vi "Dryer Start Stop.vi"() -> ()   [LabVIEW 2016]
uses:
  Type Definitions/WILT Dryer Status Ctrl.ctl
  Type Definitions/WILT Start Stop Data.ctl
  Type Definitions/WILT Dryer Com Port Info.ctl
  Globals/Globals SS.vi
  <vilib>/Utility/file.llb/Write To Spreadsheet File (string).vi
  <vilib>/DAQmx/create/channels.llb/DAQmx Create Channel (DO-Digital Output).vi
  <vilib>/DAQmx/write.llb/DAQmx Write (Digital U32 1Chan 1Samp).vi
  <vilib>/Utility/file.llb/Write To Spreadsheet File (DBL).vi
  <vilib>/DAQmx/configure/timing.llb/DAQmx Timing (Sample Clock).vi
  <vilib>/DAQmx/create/channels.llb/DAQmx Create Channel (AI-Voltage-Basic).vi
  <vilib>/Utility/file.llb/Read From Spreadsheet File (DBL).vi
  <vilib>/DAQmx/read.llb/DAQmx Read (Analog 2D DBL NChan NSamp).vi
panel:
  in  "Tab Control":T1(tab)=enum."Raw Data"
  in  "D Data 2":dbl[](array[numeric])=[0.06788055309111314, 0.06788055309111314, 0.06788055309111314, 0.06788055309111314, 0.06788055309111314, 0.06788055309111314, 0.06788055309111314, 0.06788055309111314, 0.06788055309111314, 0.06788055309111314, 0.06788055309111314, 0.06788055309111314, 0.06788055309111314, 0.06788055309111314, 0.06788055309111314]
  in  "A Data 2":dbl[](array[numeric])
  in  "A Data":dbl[](array[numeric])
  in  "B Data":dbl[](array[numeric])
  in  "B Data 2":dbl[](array[numeric])
  in  "C Data 2":dbl[](array[numeric])
  in  "C Data":dbl[](array[numeric])
  in  "D Data":dbl[](array[numeric])=[5.851428694297497, 3.661927497414327, 3.661927497414327, 3.661927497414327, 3.661927497414327, 3.661927497414327, 3.661927497414327, 3.661927497414327, 3.661927497414327, 0.6577281807606751, 0.09762322341846881, 0.09762322341846881, 0.09762322341846881, 0.09762322341846881, 0.09762322341846881]
  in  "A save":dbl[](array[numeric])
  in  "C save":dbl[](array[numeric])
  in  "B save":dbl[](array[numeric])
  in  "D save":dbl[](array[numeric])=[5.851428694297497, 3.661927497414327, 3.661927497414327, 3.661927497414327, 3.661927497414327, 3.661927497414327, 3.661927497414327, 3.661927497414327, 3.661927497414327, 0.6577281807606751, 0.09762322341846881, 0.09762322341846881, 0.09762322341846881, 0.09762322341846881, 0.09762322341846881]
  out "Waveform Chart":dbl(graph)=0.09762322341846881
  in  "Channel":i32=6
  out "Currents":dbl[](array[numeric])=[0.0012165306634386985, -0.006587335189708488, 0.00045533310115012174, 0.009590983127054642, 0.09094609304713201, 0.048033305281516, 0.09762322341846881, 0.06788055309111314] format="%0.2f"
  in  "AI Task":refnum<k21>
  in  "Maximum Value":dbl=10.0 format="%0.2f"
  in  "Minimum Value":dbl=-10.0 format="%0.2f"
  in  "Rate":dbl=2.0 caption="Sample Rate (Hz)" format="%0.2f"
  in  "Samples per Channel":i32=1
  out "data":dbl[][](array[numeric])=[[0.0002433061326877397], [-0.0013174670379416976], [9.106662023002435e-05], [0.0019181966254109284], [0.018189218609426402], [0.0096066610563032], [0.019524644683693762], [0.013576110618222628]] format="%0.2f"
  in  "AI Channel":string="Dev2/ai0:7"
  out "Current State":string="Exit"
  out "Saving":errorcluster
  out "Stop":bool=TRUE
  out "Read Serial Count":dbl=792.0
  out "Log Coms Array":string[](array[string])=["COM2,3/1/2012,10:47:12 AM,No Com", "COM3,3/1/2012,10:47:12 AM,No Com", "COM4,3/1/2012,10:47:12 AM,No Com", "COM5,3/1/2012,10:47:12 AM,"]
  out "Status Array Out":T2[](array[typedef])=[{"Color"=0, "Last Read Status"=enum."Err", "Command:Data"="No Com", "Com Port"=2, "Time(S)"=158.546875, "Err Count"=233}, {"Color"=0, "Last Read Status"=enum."Err", "Command:Data"="No Com", "Com Port"=3, "Time(S)"=158.546875, "Err Count"=233}, {"Color"=0, "Last Read Status"=enum."Err", "Command:Data"="No Com", "Com Port"=4, "Time(S)"=158.5625, "Err Count"=233}, {"Color"=6618880, "Last Read Status"=enum."Cycle Running", "Command:Data"="", "Com Port"=5, "Time(S)"=158.5625, "Err Count"=1}]
  out "Rising Edge Out":bool[](array[boolean])
  in  "Power":bool[](array[boolean])=[FALSE, FALSE, FALSE, FALSE]
  in  "Power Port":tag="Dev2/port0" caption="Port"
  out "Restart Err Count":dbl=1.0
  in  "Cycle Save Multiple":i16=25
  out "Com Er Mess":string="Send Restart"
  out "Label Com Array":string[][](array[string])=[["Dryer A", "2"], ["Dryer B", "3"], ["Dryer C", "4"], ["Dryer D", "5"]]
  out "Current Filename":path=path "C:/Data/20120301_10_CONWAY-E5500.appl.ge.com_Dryer A_SS_Data.csv"
  in  "Timeout":i32=500
  in  "Config File":path=path "C:/data/SS_Config.ini"
  in  "Save File Path":path=path "C:/Data/Start Stop"
  out "robo?":bool
  out "Computer Name":string="CONWAY-E5500.appl.ge.com"
  in  "Cycle Count Path":path=path "c:/Data/CycleCount.csv"
  in  "Backup Hour":string="4"
  in  "Up Lim":dbl[](array[numeric])=[50.0, 50.0, 50.0, 50.0, 50.0, 4.4, 4.4, 50.0, 50.0, 50.0, 50.0, 1.0, 1.0, 1.0, 50.0, 50.0, 50.0, 50.0, 50.0, 50.0, 27.0, 27.0, 27.0, 27.0, 27.0, 27.0, 27.0, 27.0, 1.0, 1.0, 1.0, 1.0]
  in  "Low Lim 2":dbl[](array[numeric])=[-1.0, -1.0, -1.0, -1.0, -1.0, 3.5, 3.5, -1.0, -1.0, -1.0, -1.0, -1.0, -1.0, -1.0, -1.0, -1.0, -1.0, -1.0, -1.0, -1.0, -1.0, -1.0, -1.0, 22.0, -1.0, -1.0, -1.0, -1.0, -1.0, -1.0, -1.0, -1.0]
  in  "Low Lim":dbl[](array[numeric])=[-1.0, -1.0, -1.0, -1.0, -1.0, 3.5, 3.5, -1.0, -1.0, -1.0, -1.0, -1.0, -1.0, -1.0, -1.0, -1.0, -1.0, -1.0, -1.0, -1.0, -1.0, -1.0, 22.0, -1.0, -1.0, -1.0, -1.0, -1.0, -1.0, -1.0, -1.0, -1.0]
  in  "Off On Threshold":dbl=1.0
  in  "Filename Currents":path=path "c:/Data/Currents.csv"
  out "Max Len":i32
  out "A Array":string[][](array[string])
  out "B Array":string[][](array[string])
  out "D Array":string[][](array[string])=[["Dryer D,COM5,3/1/2012,10:46:45 AM,0x72:0x03\r0x72:0x03\r\nInner Coil OFF\r\nOuter Coil Relay OFF\r\nMachine EOCStep ID: 0006\r\n\r\nDrum Relay OFFCF Switch:0000"], [""], [""], [""], [""], [""], [""], ["Dryer D,COM5,3/1/2012,10:46:49 AM,0x72:0x01\r0x72:0x01\r\nMachine RunElec HS - Inlet Set Point 1 : 0330\r\nElec HS - Outlet Set Point 1 : 0135\r\nElec HS - Inlet Set Point 2: 0000\r\nElec HS - Outlet Set Point 2 : 0000\r\nElec HS - Inlet Set Point 3: 0350\r\nElec HS - Outlet Set Point 3 : 0140\r\n\r\nCurrent primitive: TimeDryStep ID: 0002\r\nBase Cycle Index: 0006\r\nEst Cycle Time In Min: 0001\r\n\r\nStart Tumble\r\nTumble"], ["Dryer D,COM5,3/1/2012,10:46:49 AM,StepID:0000\r\nCWDuration:0005\r\nStartDrum\r\nReverse Tumble set for CW\r\nDrum Relay ON\r\nCF Switch:0001\r\nDrum Started Ack\r\n1022  7113  0093  0138\r\nHtr Inh = 0004"], [""], ["Dryer D,COM5,3/1/2012,10:46:50 AM,1023  7113  0093  0138"], [""], ["Dryer D,COM5,3/1/2012,10:46:51 AM,1023  7113  0093  0138"], [""], ["Dryer D,COM5,3/1/2012,10:46:52 AM,1022  7113  0093  0139\r\n\r\nHeaterOffDuration:0000\r\nTumbleStepID:0001\r\nDrum Relay OFFReverse Tumble set for CCW"], ["Dryer D,COM5,3/1/2012,10:46:53 AM,CF Switch:0000"], ["Dryer D,COM5,3/1/2012,10:46:54 AM,1020  7113  0092  0139\r\n\r\nDrum Stop Ack\r\nCW Pause Duraiton:3000\r\nTumble Pause"], ["Dryer D,COM5,3/1/2012,10:46:54 AM,1022  7113  0092  0139"], [""], ["Dryer D,COM5,3/1/2012,10:46:55 AM,1022  7113  0093  0138"], [""], ["Dryer D,COM5,3/1/2012,10:46:56 AM,1023  7113  0093  0139\r\n\r\nTumbleStepID:0002\r\nCCWDurat"], ["Dryer D,COM5,3/1/2012,10:46:57 AM,ion:0005\r\nStartDrum\r\nDrum Relay ON\r\nCF Switch:0001"], ["Dryer D,COM5,3/1/2012,10:46:57 AM,1020  7113  0093  0139\r\nDrum Started Ack"], [""], ["Dryer D,COM5,3/1/2012,10:46:59 AM,1019  7113  0093  0139\r\nHtr Inh = 0000\r\nOuter Coil ON\r\nInner Coil ON"], ["Dryer D,COM5,3/1/2012,10:46:59 AM,1023  7113  0093  0139\r\nER1-ON \r\nER2-ON"], [""], ["Dryer D,COM5,3/1/2012,10:47:00 AM,1023  7113  0093  0139\r\n\r0x72:0x03\r0x72:0x03\r\nInner Coil OFF\r\nOuter Coil"], ["Dryer D,COM5,3/1/2012,10:47:01 AM,Relay OFF\r\nMachine EOCStep ID: 0006\r\n\r\nDrum Relay OFFCF Switch:0000"], [""], [""], [""], [""], [""], [""], ["Dryer D,COM5,3/1/2012,10:47:05 AM,0x72:0x01\r0x72:0x01\r\nMachine RunElec HS - Inlet  Outlet Set Point 1 : 0135\r\nElec HS - Inlet Set Point 2: 0000\r\nElec HS - Outlet Set Point 2 : 0000\r\nElec HS - Inlet Set Point 3: 0350\r\nElec HS - Outlet Set Point 3 : 0140\r\n\r\nCurrent primitive: TimeDryStep ID: 0002\r\nBase Cycle Index: 0006\r\nEst Cycle Time In Min: 0001\r\n\r\nStart Tumble\r\nTumbleStepID:0000\r\nCWDuration:0005"], ["Dryer D,COM5,3/1/2012,10:47:05 AM,t for CW\r\nDrum Relay ON\r\nCF Switch:0001\r\nDrum Started Ack\r\n1023  7113  0093  0139\r\nHtr Inh = 0004"], [""], ["Dryer D,COM5,3/1/2012,10:47:06 AM,1019  7113  0093  0139"], ["Dryer D,COM5,3/1/2012,10:47:07 AM,0x72:0x01\r0x72:0x01"], ["Dryer D,COM5,3/1/2012,10:47:08 AM,1021  7113  0094  0138"], [""], ["Dryer D,COM5,3/1/2012,10:47:09 AM,1021  7113  0093  0139"], ["Dryer D,COM5,3/1/2012,10:47:09 AM,HeaterOffDuration:0000\r\nTum"], ["Dryer D,COM5,3/1/2012,10:47:10 AM,bleStepID:0001\r\nDrum Relay OFFReverse Tumble set for CCW\r\n1020  7113  0094  0139\r\nCF Switch:0000"], ["Dryer D,COM5,3/1/2012,10:47:10 AM,1021  7113  0094  0139\r\n\r\nDrum Stop Ack\r\nCW Pause Dur"], ["Dryer D,COM5,3/1/2012,10:47:11 AM,aiton:3000\r\nTumble Pause"], ["Dryer D,COM5,3/1/2012,10:47:12 AM,1023  7113  0094  0139"], [""]]
  out "C Array":string[][](array[string])
  out "Ready":bool=TRUE
  in  "Change Lint":bool
  out "Station D: L1 Current":waveform(dbl)[](graph)=[{"t0"=timestamp(0 s since 1904-01-01), "dt"=0.5, "Y"=[50.0, 50.0, 50.0, 50.0, 50.0, 4.4, 4.4, 50.0, 50.0, 50.0, 50.0, 1.0, 1.0, 1.0, 50.0, 50.0, 50.0, 50.0, 50.0, 50.0, 27.0, 27.0, 27.0, 27.0, 27.0, 27.0, 27.0, 27.0, 1.0, 1.0, 1.0, 1.0]}, {"t0"=timestamp(0 s since 1904-01-01), "dt"=0.5, "Y"=[-1.0, -1.0, -1.0, -1.0, -1.0, 3.5, 3.5, -1.0, -1.0, -1.0, -1.0, -1.0, -1.0, -1.0, -1.0, -1.0, -1.0, -1.0, -1.0, -1.0, -1.0, -1.0, 22.0, -1.0, -1.0, -1.0, -1.0, -1.0, -1.0, -1.0, -1.0, -1.0]}, {"t0"=timestamp(0 s since 1904-01-01), "dt"=0.5, "Y"=[5.851428694297497, 3.661927497414327, 3.661927497414327, 3.661927497414327, 3.661927497414327, 3.661927497414327, 3.661927497414327, 3.661927497414327, 3.661927497414327, 0.6577281807606751, 0.09762322341846881, 0.09762322341846881, 0.09762322341846881, 0.09762322341846881, 0.09762322341846881]}, {"t0"=timestamp(0 s since 1904-01-01), "dt"=0.5, "Y"=[0.06788055309111314, 0.06788055309111314, 0.06788055309111314, 0.06788055309111314, 0.06788055309111314, 0.06788055309111314, 0.06788055309111314, 0.06788055309111314, 0.06788055309111314, 0.06788055309111314, 0.06788055309111314, 0.06788055309111314, 0.06788055309111314, 0.06788055309111314, 0.06788055309111314]}, {"t0"=timestamp(0 s since 1904-01-01), "dt"=0.5, "Y"=[-1.0, -1.0, -1.0, -1.0, -1.0, 3.5, 3.5, -1.0, -1.0, -1.0, -1.0, -1.0, -1.0, -1.0, -1.0, -1.0, -1.0, -1.0, -1.0, -1.0, -1.0, -1.0, -1.0, 22.0, -1.0, -1.0, -1.0, -1.0, -1.0, -1.0, -1.0, -1.0]}]
  out "Station B: L1 Current":waveform(dbl)[](graph)=[{"t0"=timestamp(0 s since 1904-01-01), "dt"=0.5, "Y"=[50.0, 50.0, 50.0, 50.0, 50.0, 4.4, 4.4, 50.0, 50.0, 50.0, 50.0, 1.0, 1.0, 1.0, 50.0, 50.0, 50.0, 50.0, 50.0, 50.0, 27.0, 27.0, 27.0, 27.0, 27.0, 27.0, 27.0, 27.0, 1.0, 1.0, 1.0, 1.0]}, {"t0"=timestamp(0 s since 1904-01-01), "dt"=0.5, "Y"=[-1.0, -1.0, -1.0, -1.0, -1.0, 3.5, 3.5, -1.0, -1.0, -1.0, -1.0, -1.0, -1.0, -1.0, -1.0, -1.0, -1.0, -1.0, -1.0, -1.0, -1.0, -1.0, 22.0, -1.0, -1.0, -1.0, -1.0, -1.0, -1.0, -1.0, -1.0, -1.0]}, {"t0"=timestamp(0 s since 1904-01-01), "dt"=0.5, "Y"=[]}, {"t0"=timestamp(0 s since 1904-01-01), "dt"=0.5, "Y"=[]}, {"t0"=timestamp(0 s since 1904-01-01), "dt"=0.5, "Y"=[-1.0, -1.0, -1.0, -1.0, -1.0, 3.5, 3.5, -1.0, -1.0, -1.0, -1.0, -1.0, -1.0, -1.0, -1.0, -1.0, -1.0, -1.0, -1.0, -1.0, -1.0, -1.0, -1.0, 22.0, -1.0, -1.0, -1.0, -1.0, -1.0, -1.0, -1.0, -1.0]}]
  out "Station C: L1 Current":waveform(dbl)[](graph)=[{"t0"=timestamp(0 s since 1904-01-01), "dt"=0.5, "Y"=[50.0, 50.0, 50.0, 50.0, 50.0, 4.4, 4.4, 50.0, 50.0, 50.0, 50.0, 1.0, 1.0, 1.0, 50.0, 50.0, 50.0, 50.0, 50.0, 50.0, 27.0, 27.0, 27.0, 27.0, 27.0, 27.0, 27.0, 27.0, 1.0, 1.0, 1.0, 1.0]}, {"t0"=timestamp(0 s since 1904-01-01), "dt"=0.5, "Y"=[-1.0, -1.0, -1.0, -1.0, -1.0, 3.5, 3.5, -1.0, -1.0, -1.0, -1.0, -1.0, -1.0, -1.0, -1.0, -1.0, -1.0, -1.0, -1.0, -1.0, -1.0, -1.0, 22.0, -1.0, -1.0, -1.0, -1.0, -1.0, -1.0, -1.0, -1.0, -1.0]}, {"t0"=timestamp(0 s since 1904-01-01), "dt"=0.5, "Y"=[]}, {"t0"=timestamp(0 s since 1904-01-01), "dt"=0.5, "Y"=[]}, {"t0"=timestamp(0 s since 1904-01-01), "dt"=0.5, "Y"=[-1.0, -1.0, -1.0, -1.0, -1.0, 3.5, 3.5, -1.0, -1.0, -1.0, -1.0, -1.0, -1.0, -1.0, -1.0, -1.0, -1.0, -1.0, -1.0, -1.0, -1.0, -1.0, -1.0, 22.0, -1.0, -1.0, -1.0, -1.0, -1.0, -1.0, -1.0, -1.0]}]
  out "Station A: L1 Current":waveform(dbl)[](graph)=[{"t0"=timestamp(0 s since 1904-01-01), "dt"=0.5, "Y"=[50.0, 50.0, 50.0, 50.0, 50.0, 4.4, 4.4, 50.0, 50.0, 50.0, 50.0, 1.0, 1.0, 1.0, 50.0, 50.0, 50.0, 50.0, 50.0, 50.0, 27.0, 27.0, 27.0, 27.0, 27.0, 27.0, 27.0, 27.0, 1.0, 1.0, 1.0, 1.0]}, {"t0"=timestamp(0 s since 1904-01-01), "dt"=0.5, "Y"=[-1.0, -1.0, -1.0, -1.0, -1.0, 3.5, 3.5, -1.0, -1.0, -1.0, -1.0, -1.0, -1.0, -1.0, -1.0, -1.0, -1.0, -1.0, -1.0, -1.0, -1.0, -1.0, 22.0, -1.0, -1.0, -1.0, -1.0, -1.0, -1.0, -1.0, -1.0, -1.0]}, {"t0"=timestamp(0 s since 1904-01-01), "dt"=0.5, "Y"=[]}, {"t0"=timestamp(0 s since 1904-01-01), "dt"=0.5, "Y"=[]}, {"t0"=timestamp(0 s since 1904-01-01), "dt"=0.5, "Y"=[-1.0, -1.0, -1.0, -1.0, -1.0, 3.5, 3.5, -1.0, -1.0, -1.0, -1.0, -1.0, -1.0, -1.0, -1.0, -1.0, -1.0, -1.0, -1.0, -1.0, -1.0, -1.0, -1.0, 22.0, -1.0, -1.0, -1.0, -1.0, -1.0, -1.0, -1.0, -1.0]}]
  out "Read_ACK":bool=TRUE
  in  "Init":bool
  out "Reading":bool
  in  "Select Station":string(combo)="Dryer D"
  in  "Command:Data":string=" 7111  0087  0114\r\n\n--------------------\n1023  7111  0087  0114\r\n\n--------------------\n1023  7111  0087  0116\r\n\n--------------------\n\r\nHeaterOffDuration:0000\r\nTumbleStepID:0001\r\nDrum Relay OFFReverse Tumble set for CCW\r\n\n--------------------\nCF Switch:0000\r\n1023  7111  0087  0116\r\n\n--------------------\n\r\nDrum Stop Ack\r\nCW Pause Duraiton:3000\r\nTumble Pause\n--------------------\n1023  7111  0087  0116\r\n\n--------------------\n1023  7111  0087  0118\r\n\n--------------------\n1022  7111  0087  0118\r\n\n--------------------\n\r\nTumbleStepID:0002\r\nCCWDuration:0005\r\nStartDrum\r\nDrum Relay ON\r\nCF Switch:0001\r\n1023  7111  0087  0120\r\n\n--------------------\nDrum Started Ack\r\n\n--------------------\n1023  7111  0087  0119\r\nHtr Inh = 0000\r\nOuter Coil ON\r\nInner Coil ON\r\n\n--------------------\n1023  7111  0088  0120\r\nER1-ON \r\nER2-ON \r\n\n--------------------\n1023  7111  0088  0120\r\n\r0x72:0x03\r0x72:0x03\r\nInner Coil OFF\r\nOuter Coil \n--------------------\nRelay OFF\r\nMachine EOCStep ID: 0006\r\n\r\nDrum Relay OFFCF Switch:0000\r\n\n--------------------\n0x72:0x01\r0x72:0x01\r\nMachine RunElec HS - Inlet Set Point 1 : 0330\r\nElec HS - Outlet Set Point 1 : 0135\r\nElec HS - Inlet Set Point 2: 0000\r\nElec HS - Outlet Set Point 2 : 0000\r\nElec HS - Inlet Set Point 3: 0350\r\nElec HS - Outlet Set Point 3 : 0140\r\n\r\nCurrent primitive: TimeDryStep ID: 0002\r\nBase Cycle Index: 0006\r\nEst Cycle Time In Min: 0001\r\n\r\nStart Tumble\r\nTumble\n--------------------\nStepID:0000\r\nCWDuration:0005\r\nStartDrum\r\nReverse Tumble set for CW\r\nDrum Relay ON\r\nCF Switch:0001\r\nDrum Started Ack\r\n1022  7111  0088  0123\r\nHtr Inh = 0004\n--------------------\n1023  7111  0088  0123\r\n\n--------------------\n1023  7111  0088  0124\r\n\n--------------------\n1023  7111  0088  0124\r\n\n--------------------\n\r\nHeaterOffDuration:0000\r\nTum\n--------------------\nbleStepID:0001\r\nDrum Relay OFFReverse Tumble set for CCW\r\n1023  7111  0088  0125\r\nCF Switch:0000\r\n\n--------------------\n1023  7111  0088  0124\r\n\r\nDrum Stop Ack\r\nCW Pause Dur\n--------------------\naiton:3000\r\nTumble Pause\n--------------------\n1021  7111  0088  0125\r\n\n--------------------\n1023  7111  0088  0126\r\n\n--------------------\n1023  7111  0089  0126\r\n\r\nTumbleStepID:0002\r\nCCWDuration:0005\r\nStartDrum\r\nDrum Relay ON\r\n\n--------------------\nCF Switch:0001\r\n1023  7111  0088  0126\r\n\n--------------------\nDrum Started Ack\r\n\n--------------------\n1023  7111  0089  0126\r\nHtr Inh = 0000\r\nOuter Coil ON\r\nInner Coil ON\r\n\n--------------------\n1023  7111  0089  0127\r\nER1-ON \r\nER2-ON \r\n\n--------------------\n0x72:0x03\r0x72:0x03\r\nInner Coil OFF\r\nOuter Coil Relay OFF\r\nMachine EOCStep ID: 0006\r\n\r\nDrum Relay OFFCF Switch:0000\r\n\n--------------------\n0x72:0x01\r0x72:0x01\r\nMachine RunElec HS - Inlet Set Point 1 : 0330\r\nElec HS - Outlet Set Point 1 : 0135\r\nElec HS - Inlet Set Point 2: 0000\r\nElec HS - Outlet Set Point 2 : 0000\r\nElec HS - Inlet Set Point 3: 0350\r\nElec HS - Outlet Set Point 3 : 0140\r\n\r\nCurrent primitive: TimeDryStep ID: 0002\r\nBase Cycle Index: 0006\r\nEst Cycle Time In Min: 0001\r\n\r\nStart Tumble\r\nTumble\n--------------------\nStepID:0000\r\nCWDuration:0005\r\nStartDrum\r\nReverse Tumble set for CW\r\nDrum Relay ON\r\nCF Switch:0001\r\nDrum Started Ack\r\n1023  7111  0089  0127\r\nHtr Inh = 0004\n--------------------\n1023  7111  0089  0128\r\n\n--------------------\n1023  7111  0089  0127\r\n\n--------------------\n1023  7111  0089  0127\r\n\n--------------------\n\r\nHeaterOffDuration:0000\r\nTumbleStepID:0001\r\nDrum Relay OFFReverse Tumble set for CCW\r\n\n--------------------\nCF Switch:0000\r\n1023  7111  0089  0128\r\n\n--------------------\n\r\nDrum Stop Ack\r\nCW Pause Duraiton:3000\r\nTumble Pause1023 \n--------------------\n 7111  0090  0127\r\n\n--------------------\n1023  7111  0090  0128\r\n\n--------------------\n0x72:0x01\r0x72:0x01\n--------------------\n1023  7111  0090  0128\r\n\n--------------------\n\r\nTumbleStepID:0002\r\nCCWDuration:0005\r\nStartDrum\r\nDrum Relay ON\r\n1023  7111  0090  0128\r\n\n--------------------\nCF Switch:0001\r\n\n--------------------\nDrum Started Ack\r\n1023  7111  0090  0128\r\nHtr Inh = 0000\r\nOuter Coil ON\r\nInner Coil ON\r\n\n--------------------\n1023  7111  0090  0129\r\nER1-ON \r\nER2-ON \r\n\n--------------------\n1023  7111  0090  0128\r\n\n--------------------\n0x72:0x03\r0x72:0x03\r\nInner Coil OFF\r\nOuter Coil Relay OFF\r\nMachine EOCStep ID: 0006\r\n\r\nDrum Relay OFFCF Switch:0000\r\n\n--------------------\n0x72:0x01\r0x72:0x01\r\nMachine RunElec HS - Inlet Set Point 1 : 0330\r\nElec HS - Outlet Set Point 1 : 0135\r\nElec HS - Inlet Set Point 2: 0000\r\nElec HS - Outlet Set Point 2 : 0000\r\nElec HS - Inlet Set Point 3: 0350\r\nElec HS - Outlet Set Point 3 : 0140\r\n\r\nCurrent primitive: TimeDryStep ID: 0002\r\nBase Cycle Index: 0006\r\nEst Cycle Time In Min: 0001\r\n\r\nStart Tumble\r\nTumbleStepID:0000\r\nCWDuration:0005\r\n--------------------\n\nStartDrum\r\nReverse Tumble set for CW\r\nDrum Relay ON\r\nCF Switch:0001\r\nDrum Started Ack\r\n1023  7111  0090  0129\r\nHtr Inh = 0004\n--------------------\n1023  7111  0090  0131\r\n\n--------------------\n1023  7111  0090  0130\r\n\n--------------------\n1023  7111  0090  0131\r\n\n--------------------\n\r\nHeaterOffDuration:0000\r\nTumbleStepID:0001\r\nDrum Relay OFFReverse Tumble set for CCW\r\nCF Switch:0000\r\n1023  7111  0\n--------------------\n091  0131\r\n\n--------------------\n\r\nDrum Stop Ack\r\nCW Pause Duraiton:3000\r\nTumble Pause1023  7111  0090  0131\r\n\n--------------------\n1023  7111  0091  0132\r\n\n--------------------\n1023  7111  0091  0132\r\n\n--------------------\n\r\nTumbleStepID:0002\r\nCCWDurat\n--------------------\nion:0005\r\nStartDrum\r\nDrum Relay ON\r\n1023  7111  0091  0133\r\nCF Switch:0001\r\n\n--------------------\nDrum Started Ack\r\n1022  7111  0091  0133\r\nHtr I\n--------------------\nnh = 0000\r\nOuter Coil ON\r\nInner Coil ON\r\n\n--------------------\n1023  7111  0091  0134\r\nER1-ON \r\nER2-ON \r\n\n--------------------\n1022  7111  0091  0134\r\n\n--------------------\n0x72:0x03\r0x72:0x03\r\nInner Coil OFF\r\nOuter Coil Relay OFF\r\nMachine EOCStep ID\n--------------------\n: 0006\r\n\r\nDrum Relay OFFCF Switch:0000\r\n\n--------------------\n0x72:0x01\r0x72:0x01\r\nMachine RunElec HS - Inlet  Outlet Set Point 1 : 0135\r\nElec HS - Inlet Set Point 2: 0000\r\nElec HS - Outlet Set Point 2 : 0000\r\nElec HS - Inlet Set Point 3: 0350\r\nElec HS - Outlet Set Point 3 : 0140\r\n\r\nCurrent primitive: TimeDryStep ID: 0002\r\nBase Cycle Index: 0006\r\nEst Cycle Time In Min: 0001\r\n\r\nStart Tumble\r\nTumbleStepID:0000\r\nCWDuration:0005\r\n--------------------\n\nStartDrum\r\nReverse Tumble set for CW\r\nDrum Relay ON\r\nCF Switch:0001\r\nDrum Started Ack\r\n1023  7111  0092  0134\r\nHtr Inh = 0004\n--------------------\n1022  7111  0091  0135\r\n\n--------------------\n1022  7111  0091  0135\r\n\n--------------------\n1023  7111  0092  0135\r\n\r\nHeaterOffDuration:0000\r\nTum\n--------------------\nbleStepID:0001\r\nDrum Relay OFFReverse Tumble set for CCW\r\nCF Switch:0000\r\n1020  7111  0092  0136\r\n\n--------------------\n\r\nDrum Stop Ack\r\nCW Pause Duraiton:3000\r\nTumble Pause1021  7111  0092  0136\r\n\n--------------------\n1019  7111  0092  0136\r\n\n--------------------\n1019  7111  0091  0136\r\n\n--------------------\n\r\nTumbleStepID:0002\r\nCCWDuration:0005\r\nStartDrum\r\nDrum Relay ON\r\n\n--------------------\nCF Switch:0001\r\n1022  7111  0092  0136\r\n\n--------------------\nDrum Started Ack\r\n1023  7111  0091  0137\r\nHtr I\n--------------------\nnh = 0000\r\nOuter Coil ON\r\nInner Coil ON\r\n\n--------------------\n1023  7111  0092  0138\r\nER1-ON \r\nER2-ON \r\n\n--------------------\n1023  7111  0092  0137\r\n\n--------------------\n0x72:0x03\r0x72:0x03\r\nInner Coil OFF\r\nOuter Coil Relay OFF\r\nMachine EOCStep ID: 0006\r\n\r\nDrum Relay OFFCF Switch:0000\r\n\n--------------------\n0x72:0x01\r0x72:0x01\r\nMachine RunElec HS - Inlet Set Point 1 : 0330\r\nElec HS - Outlet Set Point 1 : 0135\r\nElec HS - Inlet Set Point 2: 0000\r\nElec HS - Outlet Set Point 2 : 0000\r\nElec HS - Inlet Set Point 3: 0350\r\nElec HS - Outlet Set Point 3 : 0140\r\n\r\nCurrent primitive: TimeDryStep ID: 0002\r\nBase Cycle Index: 0006\r\nEst Cycle Time In Min: 0001\r\n\r\nStart Tumble\r\nTumble\n--------------------\nStepID:0000\r\nCWDuration:0005\r\nStartDrum\r\nReverse Tumble set for CW\r\nDrum Relay ON\r\nCF Switch:0001\r\nDrum Started Ack\r\n1022  7113  0093  0138\r\nHtr Inh = 0004\n--------------------\n1023  7113  0093  0138\r\n\n--------------------\n1023  7113  0093  0138\r\n\n--------------------\n1022  7113  0093  0139\r\n\r\nHeaterOffDuration:0000\r\nTumbleStepID:0001\r\nDrum Relay OFFReverse Tumble set for CCW\r\n\n--------------------\nCF Switch:0000\r\n\n--------------------\n1020  7113  0092  0139\r\n\r\nDrum Stop Ack\r\nCW Pause Duraiton:3000\r\nTumble Pause\n--------------------\n1022  7113  0092  0139\r\n\n--------------------\n1022  7113  0093  0138\r\n\n--------------------\n1023  7113  0093  0139\r\n\r\nTumbleStepID:0002\r\nCCWDurat\n--------------------\nion:0005\r\nStartDrum\r\nDrum Relay ON\r\nCF Switch:0001\r\n\n--------------------\n1020  7113  0093  0139\r\nDrum Started Ack\r\n\n--------------------\n1019  7113  0093  0139\r\nHtr Inh = 0000\r\nOuter Coil ON\r\nInner Coil ON\r\n\n--------------------\n1023  7113  0093  0139\r\nER1-ON \r\nER2-ON \r\n\n--------------------\n1023  7113  0093  0139\r\n\r0x72:0x03\r0x72:0x03\r\nInner Coil OFF\r\nOuter Coil \n--------------------\nRelay OFF\r\nMachine EOCStep ID: 0006\r\n\r\nDrum Relay OFFCF Switch:0000\r\n\n--------------------\n0x72:0x01\r0x72:0x01\r\nMachine RunElec HS - Inlet  Outlet Set Point 1 : 0135\r\nElec HS - Inlet Set Point 2: 0000\r\nElec HS - Outlet Set Point 2 : 0000\r\nElec HS - Inlet Set Point 3: 0350\r\nElec HS - Outlet Set Point 3 : 0140\r\n\r\nCurrent primitive: TimeDryStep ID: 0002\r\nBase Cycle Index: 0006\r\nEst Cycle Time In Min: 0001\r\n\r\nStart Tumble\r\nTumbleStepID:0000\r\nCWDuration:0005\r\n--------------------\nt for CW\r\nDrum Relay ON\r\nCF Switch:0001\r\nDrum Started Ack\r\n1023  7113  0093  0139\r\nHtr Inh = 0004\n--------------------\n1019  7113  0093  0139\r\n\n--------------------\n0x72:0x01\r0x72:0x01\n--------------------\n1021  7113  0094  0138\r\n\n--------------------\n1021  7113  0093  0139\r\n\n--------------------\n\r\nHeaterOffDuration:0000\r\nTum\n--------------------\nbleStepID:0001\r\nDrum Relay OFFReverse Tumble set for CCW\r\n1020  7113  0094  0139\r\nCF Switch:0000\r\n\n--------------------\n1021  7113  0094  0139\r\n\r\nDrum Stop Ack\r\nCW Pause Dur\n--------------------\naiton:3000\r\nTumble Pause\n--------------------\n1023  7113  0094  0139\r\n"
  in  "UI Array":T4[](array[typedef])=[{"Label"="Dryer A", "Color"=0, "Last Read Status"=enum."Err", "Command:Data"="No Com", "Err Count"=233, "Cycle Count"=0}, {"Label"="Dryer B", "Color"=0, "Last Read Status"=enum."Err", "Command:Data"="No Com", "Err Count"=233, "Cycle Count"=0}, {"Label"="Dryer C", "Color"=0, "Last Read Status"=enum."Err", "Command:Data"="No Com", "Err Count"=233, "Cycle Count"=0}, {"Label"="Dryer D", "Color"=6618880, "Last Read Status"=enum."Cycle Running", "Command:Data"="", "Err Count"=1, "Cycle Count"=9}]
  in  "Exit":bool
  out "A Alarm":bool
  out "B Alarm":bool
  out "C Alarm":bool
  out "D Alarm":bool
  # "Used for rising edge to detect start of cycle."
  # "If after its done, the power is above this\nlimit, the contactor will remove power from the\ndryer."
  # "Restarts when 2 consec samples are < Off Limit, and Above On limit.\nSamples must be below Up Lim, and above either of the Low Lims.  Does not restart between the samples Restart LL, and Restart UL.  If after an alarm, the \ncurrent is > Off Current Lim, then shuts off power."
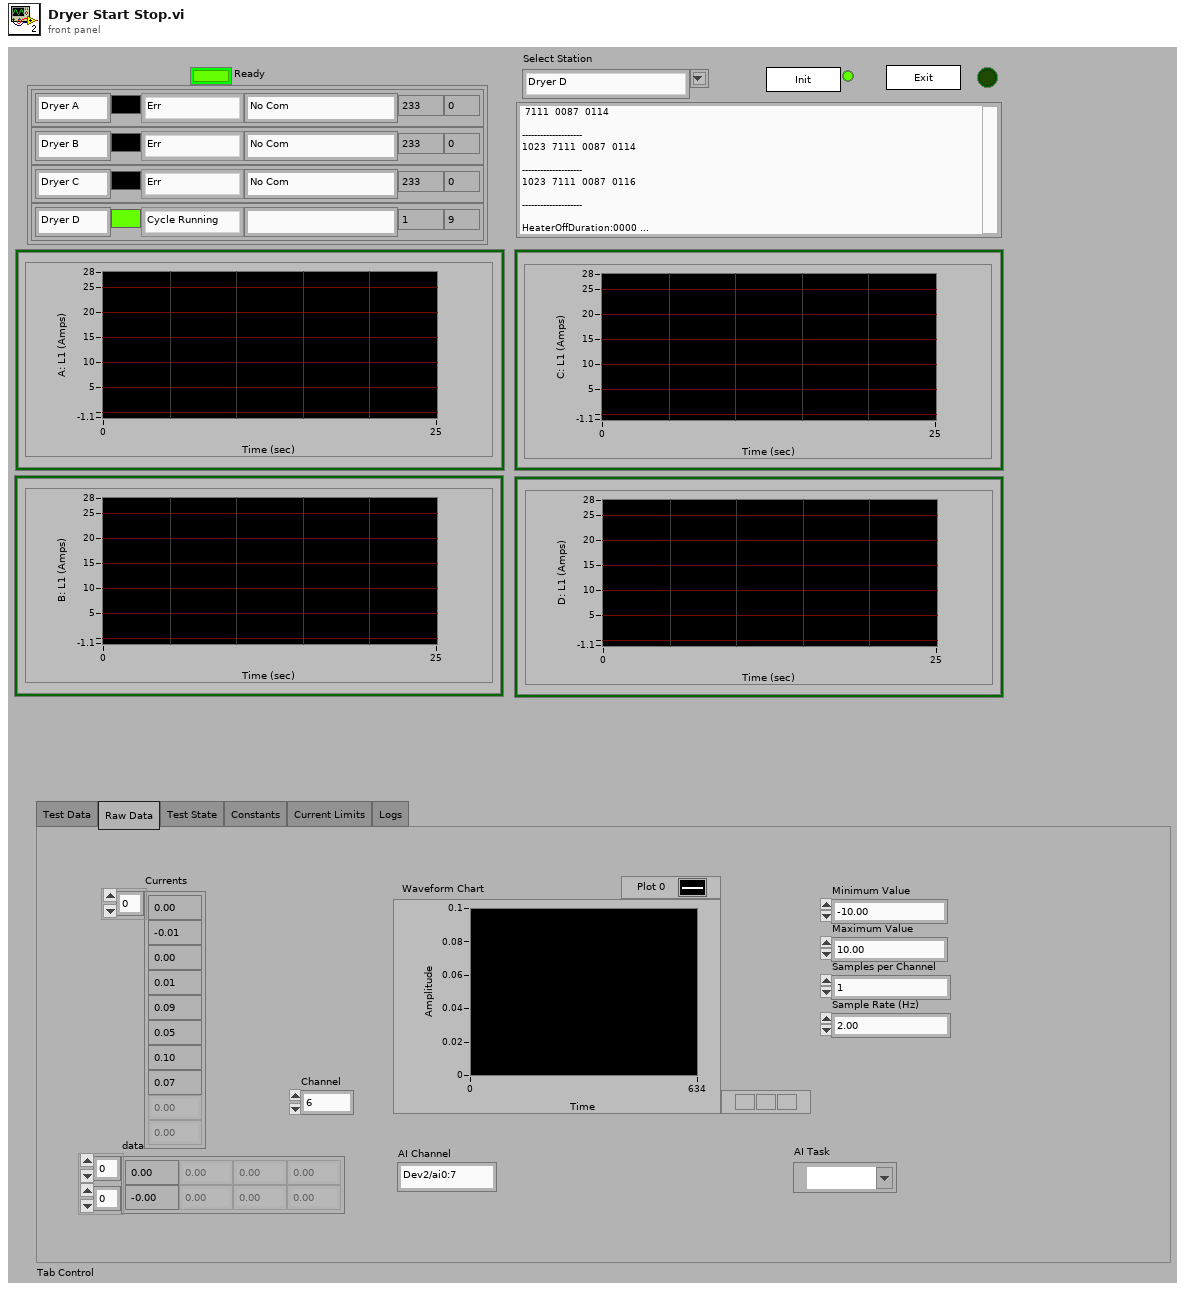
[diagram p1: front panel]
types:
  T1 = enum32{"Test Data", "Raw Data", "Test State", "Constants", "Current Limits", "Logs"}
  T2 = typedef "WILT Dryer Com Port Info.ctl" = cluster{"Color":u32, "Last Read Status":T3, "Command:Data":string, "Com Port":u8, "Time(S)":dbl, "Err Count":u32}
  T3 = typedef "WILT Dryer Status Ctrl.ctl" = enum16{"Cycle Not Started", "Cycle Running", "Paused", "Cycle Completed", "Eval Mode Entered", "Err", "Pause (No GEA2)"}
  T4 = typedef "WILT Start Stop Data.ctl" = cluster{"Label":string, "Color":u32, "Last Read Status":T3, "Command:Data":string, "Err Count":u32, "Cycle Count":u32}
  T5 = enum32{"invalid app kind", "Development System", "Run Time System", "Student Edition", "Embedded LabVIEW", "Evaluation", "Custom"}
  T6 = enum32{"Invalid", "Standard", "Closed", "Hidden", "Minimized", "Maximized"}
  T7 = cluster{"Core":cluster{"Current VI Reference":refnum<vi>, "Close Panel on Exit?":bool}, "Data to Save":string[][], "Label Com Array":string[][], "UI Array":T4[], "Com Array":u8[], "Save File Path":path, "Last Hour":string, "Computer Name":string, "task out":refnum<k21>, "Power":bool[]}
  T8 = cluster{"Current VI Reference":refnum<vi>, "Close Panel on Exit?":bool}
  T9 = cluster{"A Alarm":bool, "B Alarm":bool, "C Alarm":bool, "D Alarm":bool}
  T10 = cluster{"Waveform":dbl, "Waveform":dbl, "Waveform":dbl, "Waveform":dbl}
  T11 = cluster{"Alatch":bool, "Blatch":bool, "Clatch":bool, "Dlatch":bool, "AI Task":refnum<k21>, "A Data":dbl[], "A Data2":dbl[], "B Data":dbl[], "B Data2":dbl[], "C Data":dbl[], "C Data2":dbl[], "D Data":dbl[], "D Data2":dbl[], "Read Data":dbl[], "Old Data":dbl[], "Rise":bool[]}
  T12 = cluster{"Rise[0]":bool, "Rise[1]":bool, "Rise[2]":bool, "Rise[3]":bool}
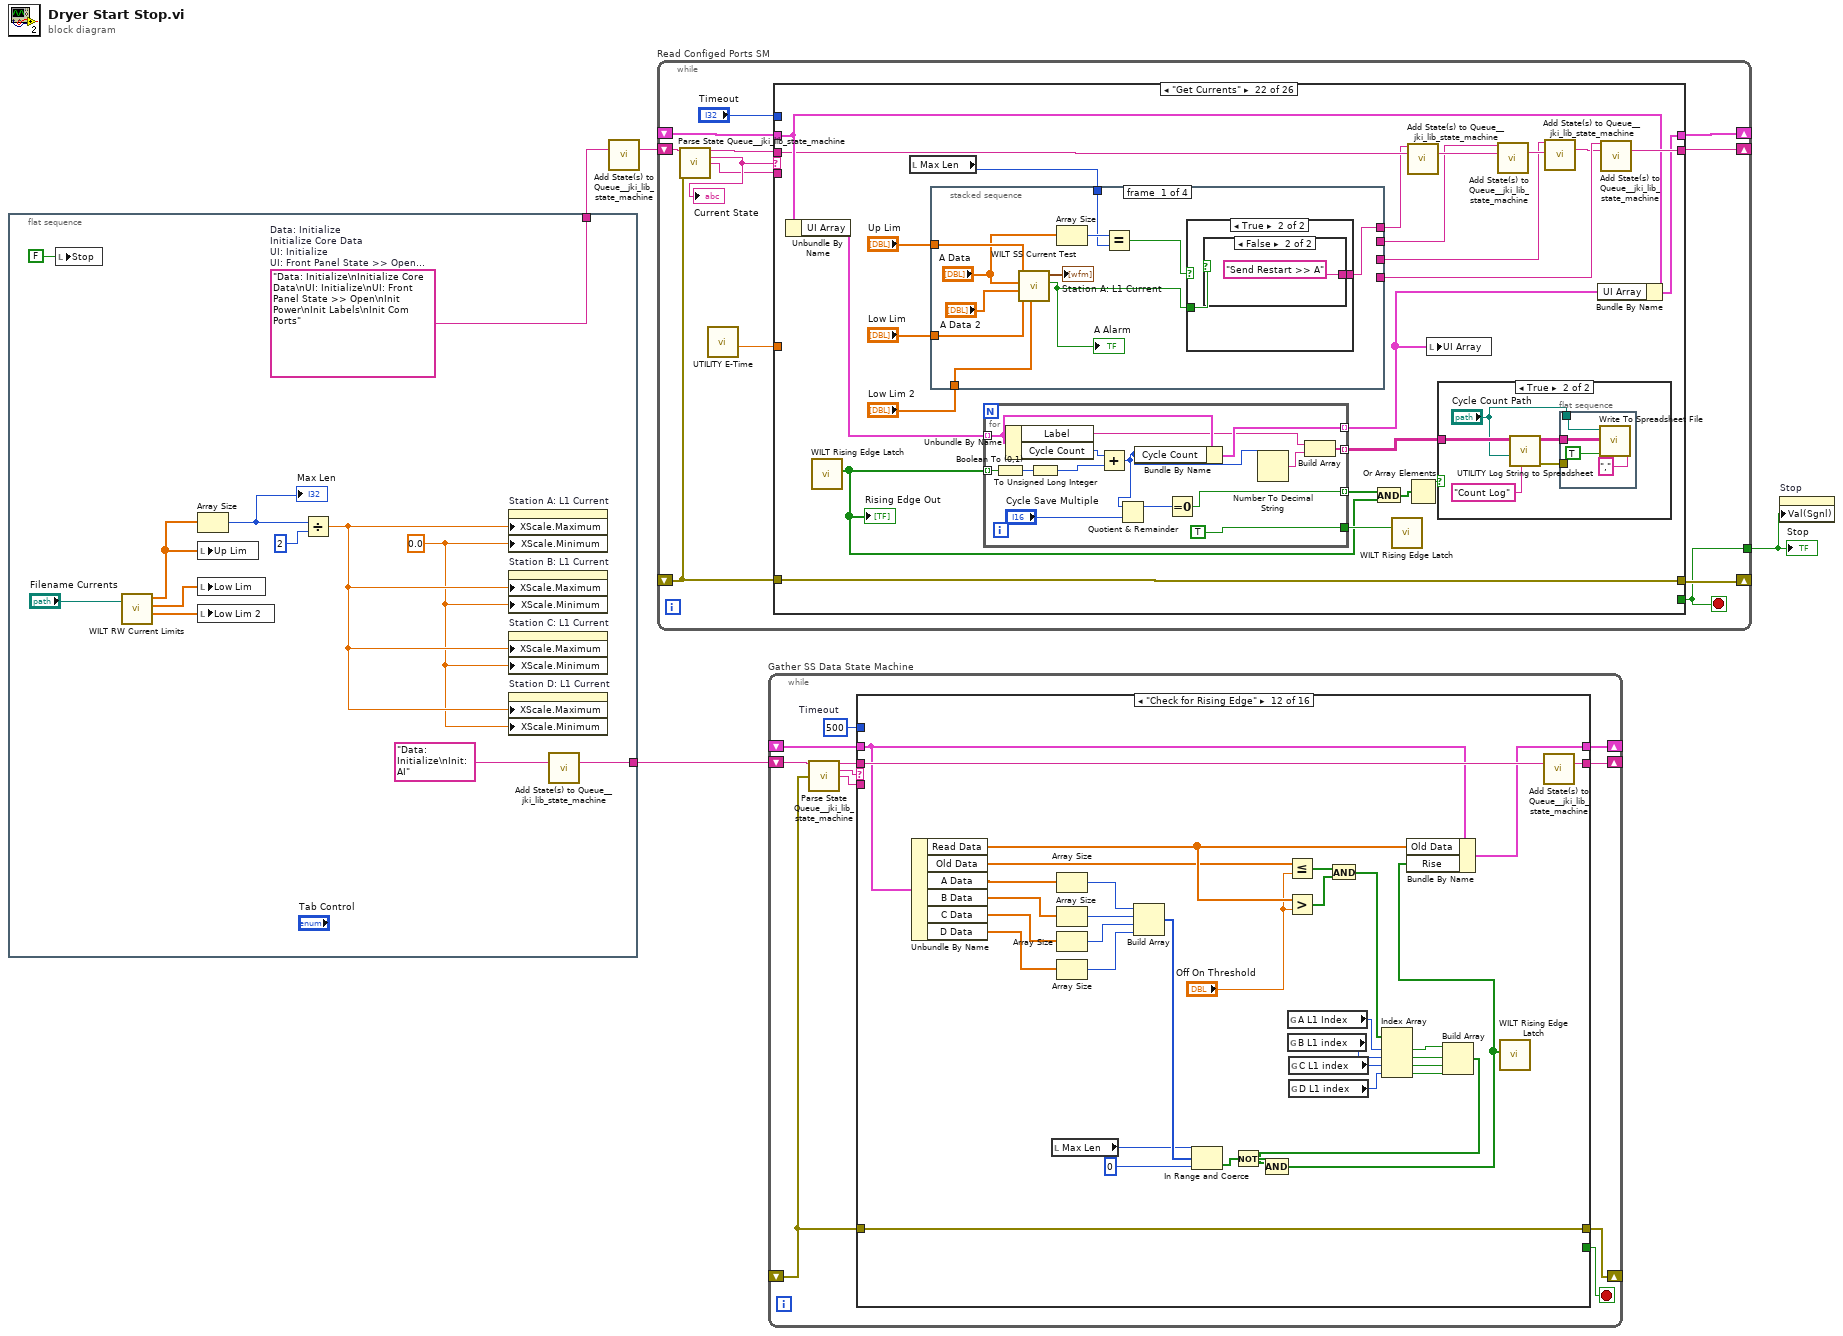
[diagram p0: block diagram]
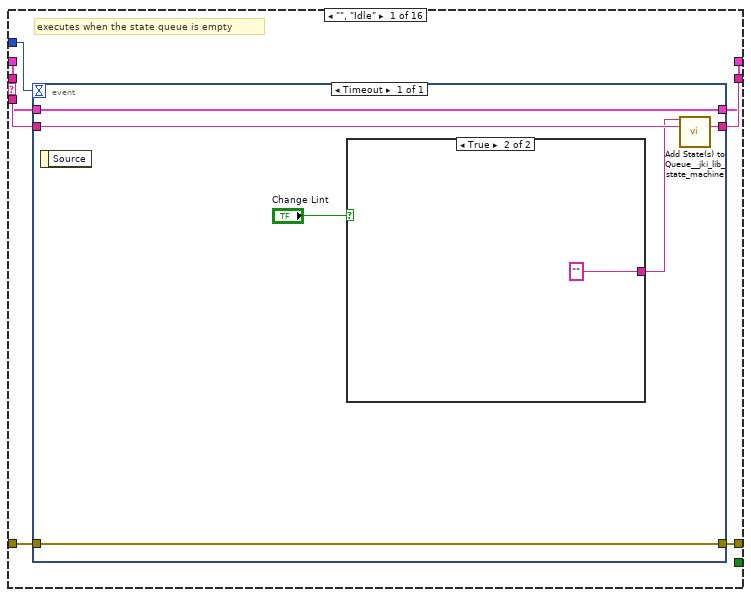
[diagram p2: hidden frame]
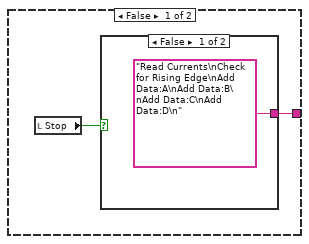
[diagram p3: hidden frame]
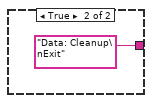
[diagram p4: hidden frame]
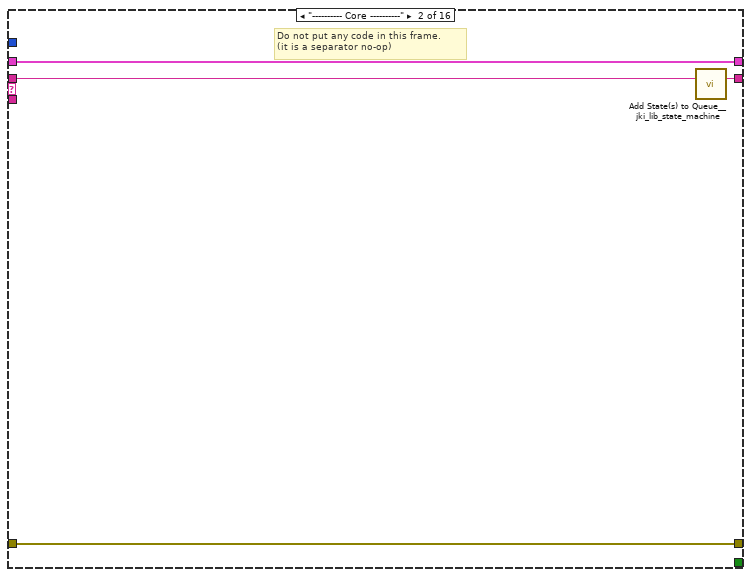
[diagram p5: hidden frame]
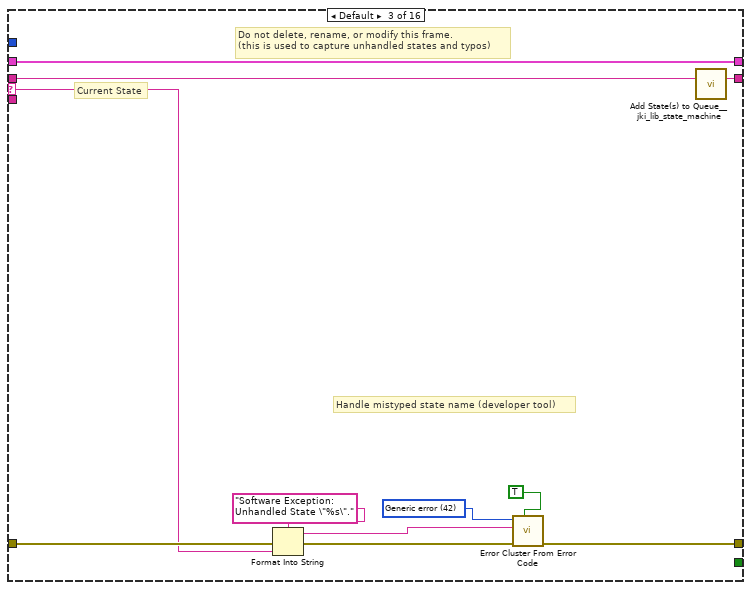
[diagram p6: hidden frame]
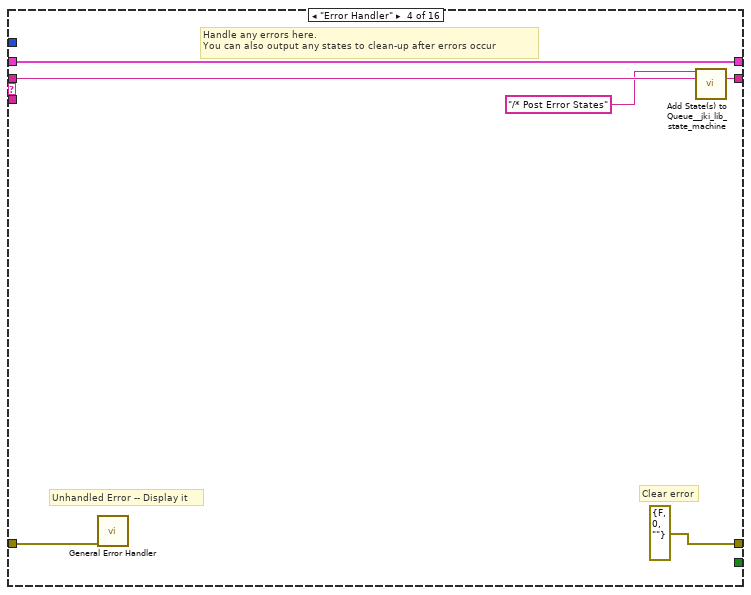
[diagram p7: hidden frame]
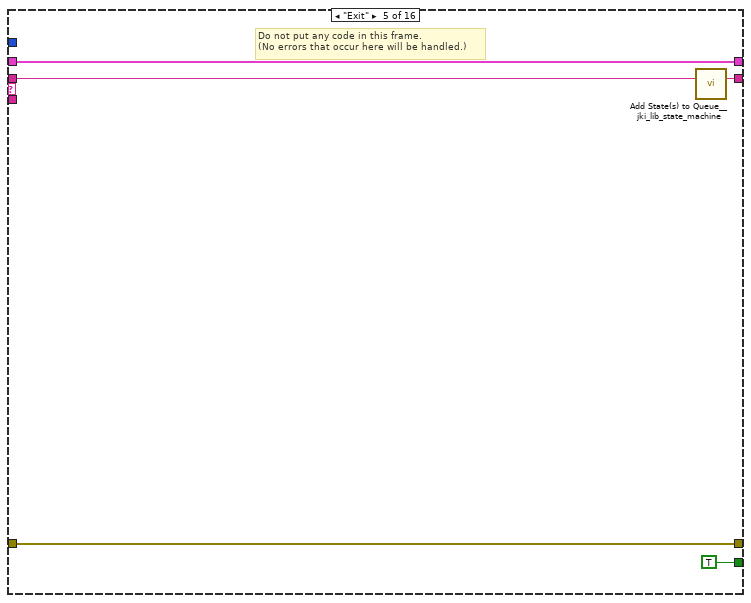
[diagram p8: hidden frame]
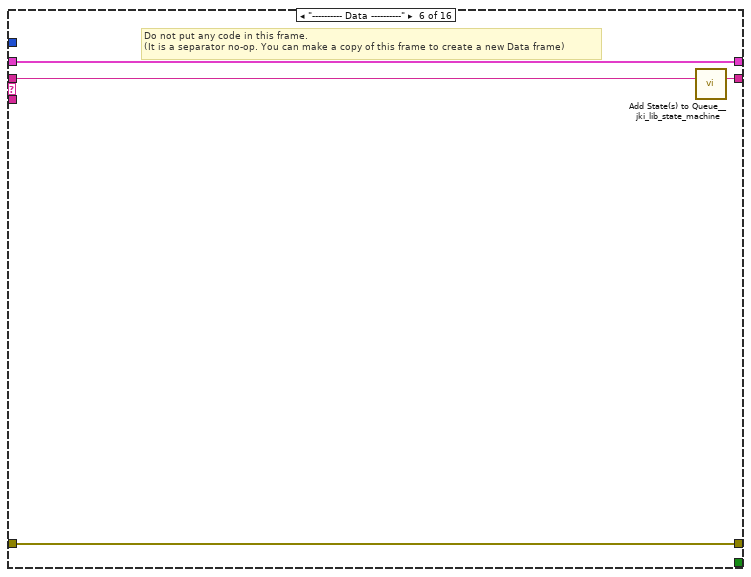
[diagram p9: hidden frame]
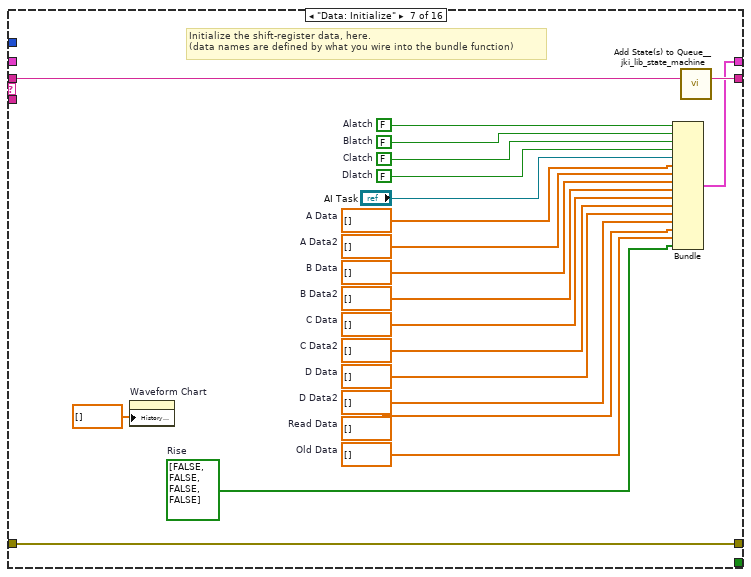
[diagram p10: hidden frame]
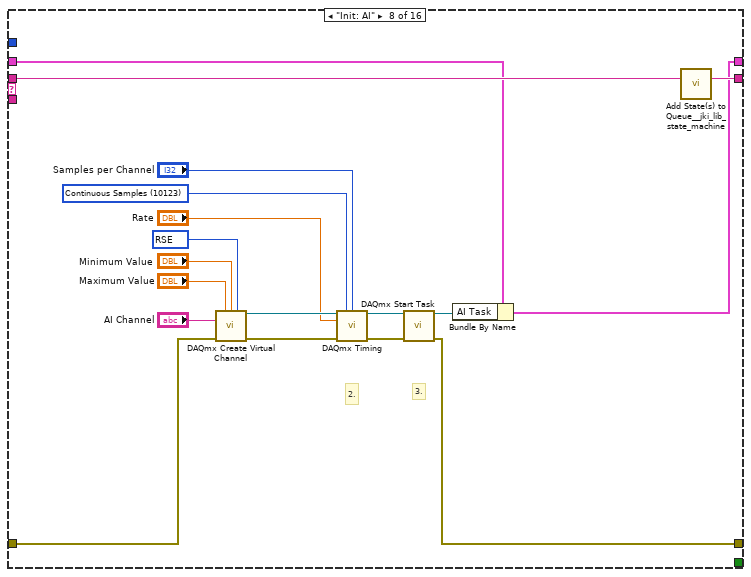
[diagram p11: hidden frame]
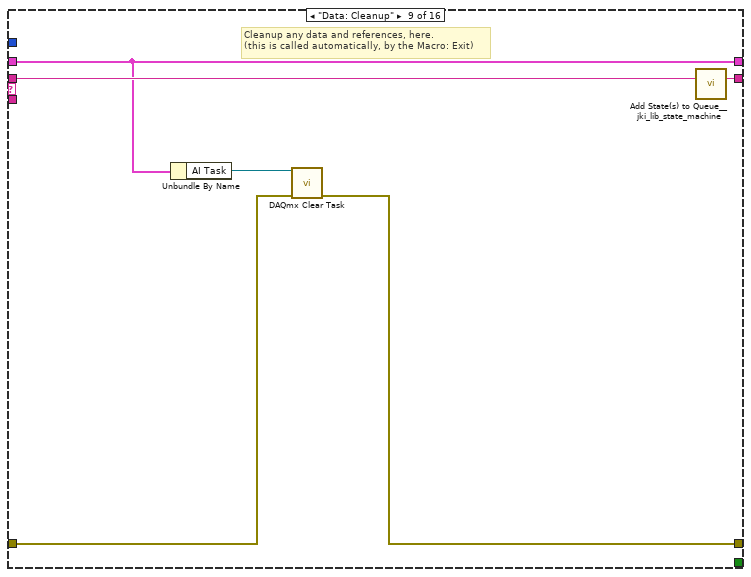
[diagram p12: hidden frame]
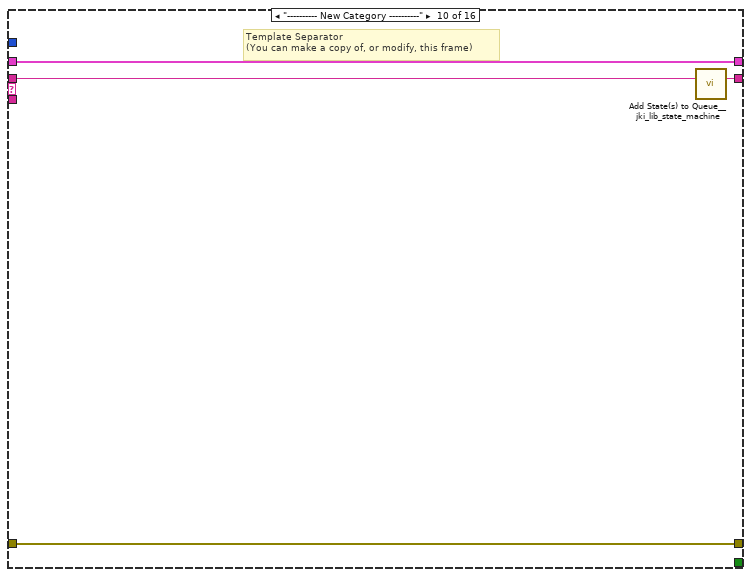
[diagram p13: hidden frame]
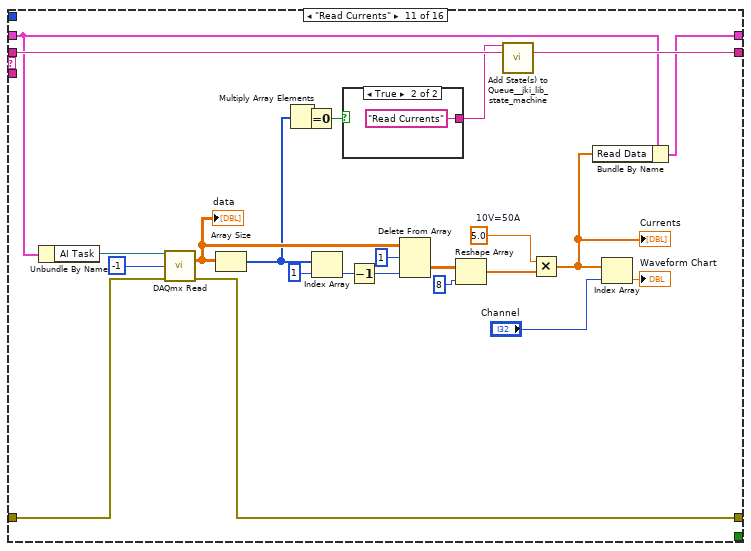
[diagram p14: hidden frame]
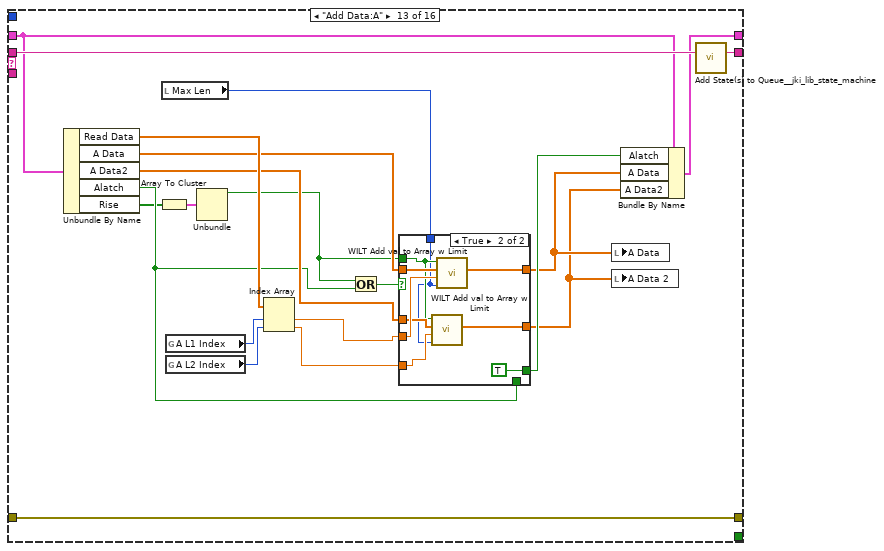
[diagram p16: hidden frame]
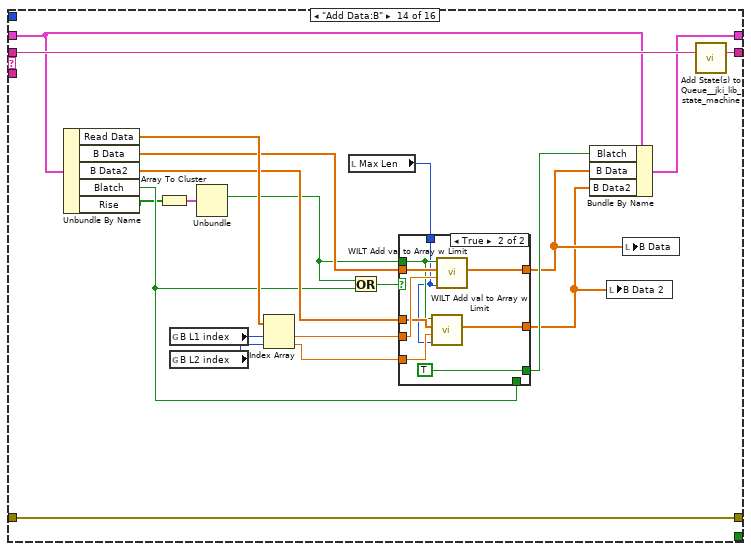
[diagram p18: hidden frame]
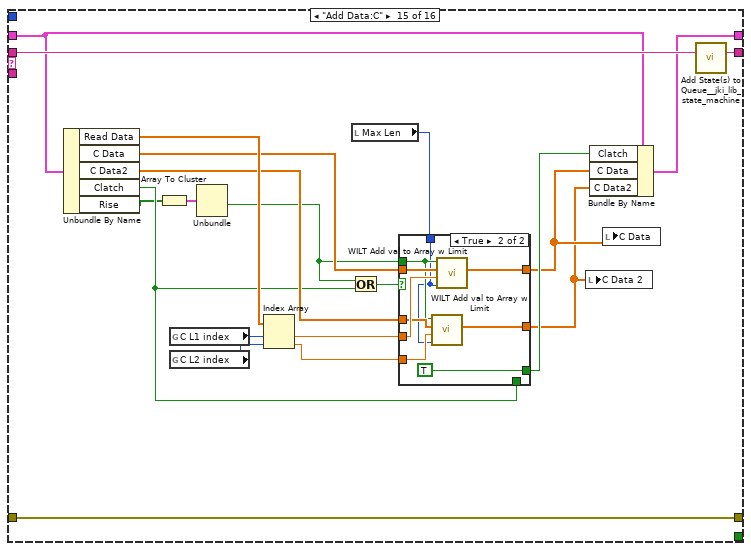
[diagram p20: hidden frame]
diagram:
  n1 = flat-sequence {
    tunnel: [w16] -> w2
    tunnel: [w15] -> w1
    frame #0 {
      w5 = 0.0 ("X Scale.Range:Minimum")
      w16 = "Data: Initialize\nInitialize Core Data\nUI: Initialize\nUI: Front Panel State >> Open\nInit Power\nInit Labels\nInit Com Ports"  # Data: Initialize Initialize Core Data UI: Initialize UI: Front Panel State >> Open Init Power Init Labels Init Com Ports
      n2 = local write "Stop"(FALSE ("Stop")) -> ()
      n3 = call "WILT RW Current Limits.vi"("file path (dialog if empty)"="Filename Currents") -> ("Low Lim 2 Out"=w10:dbl[], "Low Lim Out"=w11:dbl[], "Up Lim Out"=w9:dbl[])  [unwired: 8 in]
      n4 = Array Size(array=w9) -> (size(s)=w8:i32)
      "Max Len" <- w8
      n5 = local write "Up Lim"(w9) -> ()
      n6 = local write "Low Lim"(w11) -> ()
      n7 = local write "Low Lim 2"(w10) -> ()
      n8 = Divide(x=w8, y=2) -> (x/y=w6:dbl)
      n9 = property on="Station A: L1 Current" class="WFChart (strict)"("XScale.Maximum"=w6, "XScale.Minimum"=w5) -> ()  [unwired: 2 in, 2 out]
      n10 = property on="Station B: L1 Current" class="WFChart (strict)"("XScale.Maximum"=w6, "XScale.Minimum"=w5) -> ()  [unwired: 2 in, 2 out]
      n11 = property on="Station C: L1 Current" class="WFChart (strict)"("XScale.Maximum"=w6, "XScale.Minimum"=w5) -> ()  [unwired: 2 in, 2 out]
      n12 = property on="Station D: L1 Current" class="WFChart (strict)"("XScale.Maximum"=w6, "XScale.Minimum"=w5) -> ()  [unwired: 2 in, 2 out]
      n13 = call <vilib>:"Add State(s) to Queue__jki_lib_state_machine.vi"("State(s) in (\"\")"="Data: Initialize\nInit: AI") -> ("States Out"=w15:string)  [unwired: 14 in]
    }
  }
  n14 = call <vilib>:"Add State(s) to Queue__jki_lib_state_machine.vi"("State(s) in (\"\")"=w2) -> ("States Out"=w4:string)  [unwired: 14 in]
  n15 = while "Read Configed Ports SM" {
    shift-right: [w22] -> _
    shift-left: _ -> [w21]
    shift-right: [w24] -> _
    shift-left: _ -> [w19]
    shift-right: [w23] -> _
    shift-left: w4 -> [w25]
    tunnel: [w18] -> w3
    stop <- w18 stop-if-true
    n16 = call <vilib>:"Parse State Queue__jki_lib_state_machine.vi"("State Queue"=w25, "Error In (no error)"=w19) -> ("Remaining States"=w27:string, "Current State"=w28:string, "Arguments"=w26:string)  [unwired: 11 in]
    "Current State" <- w28
    n17 = call "UTILITY E-Time.vi"() -> ("Elapsed Time (sec)"=w17:dbl)  [unwired: 9 in, 2 out]
    n18 = case shown="\"Get Currents\"" w28 {
      selector: w28 -> [_ _ w72 _ _ _ _ _ _ _ _ w199 _ _ w244 _ _ _ _ _ _ _ _ _ _ _]
      tunnel: w27 -> [w35 w71 w76 w94 w100 w110 w114 w138 w149 w153 w178 w206 w225 w237 w248 w266 w277 w303 w308 w318 w322 w335 w459 w481 w545 w616]
      tunnel: w26 -> [_ _ _ _ _ _ _ _ _ _ _ _ _ _ w243 w261 w271 _ _ _ _ _ _ _ w513 _]
      tunnel: w21 -> [w33 w68 w74 w85 w97 w108 w111 _ w144 w150 w175 w204 w218 w234 w246 w264 w273 w300 w305 w315 w319 w342 w470 w477 w542 w613]
      tunnel: [w32 w69 w78 w91 errorcluster {"status"=FALSE, "code"=0, "source"=""} ("error out") w107 w112 w118 w145 w151 w176 w201 w222 w230 w239 w262 w274 w301 w306 w316 w320 w345 w471 w479 w543 w614] -> w24
      tunnel: w19 -> [w31 w69 w77 w91 w96 w107 w112 w119 w146 w151 w176 w202 w223 w230 w238 w263 w275 w301 w306 w316 w320 w345 w471 w479 w543 w614]
      tunnel: [w34 w70 w75 w93 w99 w109 w113 w137 w148 w152 w177 w205 w224 w236 w247 w265 w276 w302 w307 w317 w321 w346 w460 w480 w544 w615] -> w23
      tunnel: [_ _ _ _ _ TRUE _ _ _ _ _ _ _ _ _ _ _ _ _ _ _ _ _ _ _ _] -> w18
      tunnel: [w30 w68 w74 w92 w97 w108 w111 w136 w144 w150 w174 w204 w218 w233 w246 w264 w273 w300 w305 w315 w319 w341 w469 w476 w541 w613] -> w22
      tunnel: "Timeout" -> [w29 _ _ _ _ _ _ _ _ _ _ _ _ _ _ _ _ _ _ _ _ _ _ _ _ _]
      tunnel: w17 -> [_ _ _ _ _ _ _ _ _ _ _ _ _ _ _ _ _ _ _ _ _ _ _ _ _ _]
      frame "", "Idle" {
        # "executes when the state queue is empty"
        n19 = event shown="[0] Timeout" {
          selector: _ -> [_ _ _ _ _]
          dyn-events: _ -> [_ _ _ _ _]
          timeout: w29 -> [_ _ _ _ _]
          tunnel: w35 -> [w40 w43 w50 w61 w67]
          tunnel: [w39 w43 w50 w60 w66] -> w34
          tunnel: w33 -> [w37 w42 w46 w58 w64]
          tunnel: [w38 w41 w49 w59 w65] -> w32
          tunnel: w31 -> [w38 w41 w49 w59 w65]
          tunnel: [w37 w42 w46 w58 w64] -> w30
          event Timeout {
            n20 = event-data() -> ()  [unwired: 1 in, 1 out]
            n21 = call <vilib>:"Add State(s) to Queue__jki_lib_state_machine.vi"("State(s) in Front (\"\")"="Read\nGet Currents\nAdd Select Data\nCheck Power" ("State(s) in Front (\"\")"), "State(s) in (\"\")"=w40) -> ("States Out"=w39:string)  [unwired: 13 in]
          }
          event "Select Station": Value Change {
            n22 = event-data() -> ()  [unwired: 1 in, 6 out]
            n23 = local write "Command:Data"("" ("Command:Data")) -> ()
          }
          event "Init": Value Change {
            (unwired) u8 128  # Tester Source Address
            (unwired) u8 36  # Dryer Destination Address
            # "Send Command"
            n24 = event-data() -> ()  [unwired: 1 in, 6 out]
            n25 = Unbundle By Name(w46) -> ("Com Array"=w48:u8[], "Label Com Array"=w47:string[][])
            n26 = for {
              tunnel: w47 -> [w56] mode=indexing
              tunnel: w48 -> [w51] mode=indexing
              tunnel: [w51] -> w45
              stop <- w53 stop-if-true
              n27 = local read "Select Station"() -> (w52:string)
              n28 = Index Array(array=w56, index=0) -> (element=w54:string)
              n29 = Equal?(x=w54, y=w52) -> (x = y?=w53:bool)
            }
            n30 = call "UTILITY Com Chan Type Conversion.vi"("Com Chan"=w45) -> ()  [unwired: 11 in, 4 out]
          }
          event "Exit": Value Change {
            n31 = event-data() -> ()  [unwired: 1 in, 1 out]
            n32 = call <vilib>:"Add State(s) to Queue__jki_lib_state_machine.vi"("State(s) in Front (\"\")"="Macro: Exit", "State(s) in (\"\")"=w61) -> ("States Out"=w60:string)  [unwired: 13 in]
          }
          event Panel Close? {
            # "Discard the event because we'll close the front panel ourselves in Macro: Exit"
            # "Close Panel button (pressed) Event\n(this executes Macro: Exit to terminate the VI)"
            n33 = event-data() -> ()  [unwired: 1 in, 1 out]
            n34 = event-data("Discard?"=TRUE) -> ()  [unwired: 1 in, 1 out]
            n35 = call <vilib>:"Add State(s) to Queue__jki_lib_state_machine.vi"("State(s) in Front (\"\")"="Macro: Exit", "State(s) in (\"\")"=w67) -> ("States Out"=w66:string)  [unwired: 13 in]
          }
        }
      }
      frame "---------- Core ----------" {
        # "Do not put any code in this frame.\n(it is a separator no-op)"
        n36 = call <vilib>:"Add State(s) to Queue__jki_lib_state_machine.vi"("State(s) in (\"\")"=w71) -> ("States Out"=w70:string)  [unwired: 14 in]
      }
      frame Default {
        w81 = 42 items=["No error", "Argument error", "Memory is full", "Out of zone", "End of file", "File already open", "Generic file I/O error", "File not found", "File permission error", "Disk is full", "Duplicate path", "Too many files open", "System feature not enabled", "Resource file not found", "Cannot add resource", "Resource not found", "Image not found", "Image memory error", "Pen does not exist", "Config type invalid", "Config token not found", "Config parse error", "Config memory error", "Bad external code format", "Bad external code offset", "External code not present", "Null window", "Destroy window error", "Null menu", "Print aborted", "Bad print record", "Print driver error", "Windows error during printing", "Memory error during printing", "Print dialog error", "Generic print error", "Invalid device refnum", "Device not found", "Device parameter error", "Device unit error", "Cannot open device", "Device call aborted", "Generic error", "Cancelled by user", "Object ID too low", "Object ID too high", "Object not in heap", "Unknown heap", "Unknown object (invalid DefProc)", "Unknown object (DefProc not in table)", "Message out of range", "Invalid (null) method", "Unknown message", "Manager call not supported", "Bad address", "Network operation in progress", "Network operation timed out", "Connection is busy", "Network attribute not supported", "Network error", "Address in use", "System out of memory", "Connection aborted", "Connection refused", "Not connected", "Already connected", "Connection closed", "Initialization error (interapplication manager)", "Bad occurrence", "Wait on unbound occurrence handler", "Occurrence queue overflow", "Datalog type conflict", "Unused", "Unrecognized type (interapplication manager)", "Memory corrupt", "Failed to make temporary DLL", "Old CIN version", "Drag socket not found", "Failed to load drop-object", "Failed to register OLE object", "Failed to release OLE object", "Format specifier type mismatch", "Unknown format specifier", "Too few format specifiers", "Too many format specifiers", "Scan failed", "Newer CIN version", "Error converting to variant", "Runtime menu error", "Password tampered", "Variant attribute not found", "Incompatible variant data type", "Event data is not available", "Event Store is not present", "Occurrence is not found", "Event Queue is not created", "Event info is not available", "Refnum passed is NULL", "Error retrieving Class GUID", "Error retrieving CoClass GUID", "Error retrieving TypeLib GUID.", "Bad built application magic bytes.", "Specific driver is different from the specific driver associated with the Logical Name.", "There is no session opened to the class driver.", "Max Error", "MAX - Error with config objects", "MAX - Error loading configuration", "MAX - Group not supported"]
        # "Current State"
        # "Do not delete, rename, or modify this frame.\n(this is used to capture unhandled states and typos)"
        # "Handle mistyped state name (developer tool)"
        n37 = Format Into String(format string="Software Exception: Unhandled State \"%s\"." ("message"), error in=w77, w72) -> (resulting string=w80:string, error out=w79:errorcluster)  [unwired: 1 in]
        n38 = call <vilib>:"Error Cluster From Error Code.vi"("show call chain? (False)"=TRUE, "error in (no error)"=w79, "error message (\"\")"=w80, "error code (0)"=w81) -> ("error out"=w78:errorcluster)  [unwired: 5 in]
        n39 = call <vilib>:"Add State(s) to Queue__jki_lib_state_machine.vi"("State(s) in (\"\")"=w76) -> ("States Out"=w75:string)  [unwired: 14 in]
      }
      frame "Initialize Core Data" {
        # "Do not delete, rename, or modify this frame.\n(this is used to determine panel behavior on exit)"
        # "originally closed?"
        # "exe?"
        # "If panel starts closed or is an EXE, then close it when we exit"
        n40 = property class="VI"() -> ("Front Panel.Open"=w90:bool)  [unwired: 2 in, 2 out]
        n41 = property class="App"() -> ("App.Kind"=w89:T5)  [unwired: 2 in, 2 out]
        n42 = control-ref of="Current VI Reference"() -> (w83:refnum<vi>)
        n43 = Not(x=w90) -> (.not. x?=w87:bool)
        n44 = Equal?(x=w89, y=T5."Run Time System" ("Application:Kind")) -> (x = y?=w86:bool)
        n45 = Or(x=w87, y=w86) -> (x .or. y?=w84:bool)
        n46 = Bundle By Name(cluster=w85, "Core.Current VI Reference"=w83, "Core.Close Panel on Exit?"=w84) -> (w92:T7)
        n47 = call <vilib>:"Add State(s) to Queue__jki_lib_state_machine.vi"("State(s) in (\"\")"=w94) -> ("States Out"=w93:string)  [unwired: 14 in]
      }
      frame "Error Handler" {
        # "Unhandled Error -- Display it"
        # "Handle any errors here.\nYou can also output any states to clean-up after errors occur"
        # "Clear error"
        n48 = call <vilib>:"General Error Handler.vi"("error in (no error)"=w96) -> ()  [unwired: 10 in, 5 out]
        n49 = call <vilib>:"Add State(s) to Queue__jki_lib_state_machine.vi"("State(s) in Front (\"\")"="/* Post Error States", "State(s) in (\"\")"=w100) -> ("States Out"=w99:string)  [unwired: 13 in]
      }
      frame "Exit" {
        # "Do not put any code in this frame.\n(No errors that occur here will be handled.)"
        n50 = local read "Filename Currents"() -> (w101:path)
        n51 = local read "Low Lim 2"() -> (w103:dbl[])
        n52 = local read "Up Lim"() -> (w105:dbl[])
        n53 = local read "Low Lim"() -> (w104:dbl[])
        n54 = call "WILT RW Current Limits.vi"("Write?"=TRUE, "Low Lim 2"=w103, "Low Lim"=w104, "Up Lim"=w105, "file path (dialog if empty)"=w101) -> ()  [unwired: 4 in, 3 out]
        n55 = call <vilib>:"Add State(s) to Queue__jki_lib_state_machine.vi"("State(s) in (\"\")"=w110) -> ("States Out"=w109:string)  [unwired: 14 in]
      }
      frame "---------- Data ----------" {
        # "Do not put any code in this frame.\n(It is a separator no-op. You can make a copy of this frame to create a new Data frame)"
        n56 = call <vilib>:"Add State(s) to Queue__jki_lib_state_machine.vi"("State(s) in (\"\")"=w114) -> ("States Out"=w113:string)  [unwired: 14 in]
      }
      frame "Data: Initialize" {
        w122 = 1 items=["one channel for each line", "one channel for all lines"] ("line grouping")
        w125 = ""  # Last Hour
        w127 = string[][] []  # Data to Save
        w130 = u8[] []  # Com Array
        w135 = T8 {"Current VI Reference"=refnum, "Close Panel on Exit?"=FALSE}  # Core
        # "Initialize the shift-register data, here.\n(data names are defined by what you wire into the bundle function)"
        n57 = stacked-sequence {
          frame #0 {
            w139 = FALSE ("A Alarm")
            n58 = local write "A Alarm"(w139) -> ()
            n59 = local write "B Alarm"(w139) -> ()
            n60 = local write "C Alarm"(w139) -> ()
            n61 = local write "D Alarm"(w139) -> ()
            n62 = local write "Ready"(w139) -> ()
          }
          frame #1 {
            w140 = string[][] []  # Data to Save
            n63 = local write "D Array"(w140) -> ()
            n64 = local write "C Array"(w140) -> ()
            n65 = local write "A Array"(w140) -> ()
            n66 = local write "B Array"(w140) -> ()
          }
          frame #2 {
            w141 = dbl[] [] ("D Data")
            n67 = local write "C Data"(w141) -> ()
            n68 = local write "A Data"(w141) -> ()
            n69 = local write "B Data"(w141) -> ()
            n70 = local write "D Data"(w141) -> ()
            n71 = local write "C Data 2"(w141) -> ()
            n72 = local write "D Data 2"(w141) -> ()
            n73 = local write "A Data 2"(w141) -> ()
            n74 = local write "B Data 2"(w141) -> ()
          }
        }
        n75 = call "WILT Rising Edge Latch.vi"("Reset"=TRUE) -> ()  [unwired: 10 in, 1 out]
        n76 = call "WILT Read From Spreadsheet File (string) with Prompt.vi"("delimiter (\\t)"="," ("delimiter (\\t)"), "prompt"="Choose config file to read.", "file path (dialog if empty)"="Config File") -> ("all rows"=w133:string[][])  [unwired: 4 in, 4 out]
        n77 = flat-sequence {
          tunnel: w133 -> [w142]
          tunnel: [w143] -> w132
          frame #0 {
            "Label Com Array" <- w142
          }
          frame #1 {
            n78 = local read "Label Com Array"() -> (w143:string[][])
          }
        }
        n79 = call "UTILITY IP and Computer Name.vi"() -> ("Computer Name"=w123:string)  [unwired: 10 in, 1 out]
        "Computer Name" <- w123
        n80 = local write "Command:Data"(w125) -> ()
        n81 = call-poly <vilib>:"DAQmx Create Virtual Channel.vi"("lines"="Power Port", "line grouping"=w122, "error in"=w119) -> ("task out"=w120:refnum<k21>, "error out"=w121:errorcluster)  [unwired: 11 in]
        n82 = call <vilib>:"DAQmx Start Task.vi"("task/channels in"=w120, "error in"=w121) -> ("task out"=w116:refnum<k21>, "error out"=w118:errorcluster)  [unwired: 12 in]
        n83 = call <vilib>:"Add State(s) to Queue__jki_lib_state_machine.vi"("State(s) in (\"\")"=w138) -> ("States Out"=w137:string)  [unwired: 14 in]
        n84 = Bundle("Core"=w135, "Data to Save"=w127, "Label Com Array"=w132, "UI Array"="UI Array", "Com Array"=w130, "Save File Path"="Save File Path", "Last Hour"=w125, "Computer Name"=w123, "task out"=w116, "Power"="Power") -> (w136:T7)  [unwired: 1 in]
      }
      frame "Data: Cleanup" {
        # "Cleanup any data and references, here.\n(this is called automatically, by the Macro: Exit)"
        n85 = Unbundle By Name(w144) -> ("Core.Current VI Reference"=w147:refnum<vi>)
        n86 = Close Reference(reference=w147, error in (no error)=w146) -> (error out=w145:errorcluster)
        n87 = call <vilib>:"Add State(s) to Queue__jki_lib_state_machine.vi"("State(s) in (\"\")"=w149) -> ("States Out"=w148:string)  [unwired: 14 in]
      }
      frame "---------- UI ----------" {
        # "Do not put any code in this frame.\n(It is a separator no-op. You can make a copy of this frame to create a new UI frame)"
        n88 = call <vilib>:"Add State(s) to Queue__jki_lib_state_machine.vi"("State(s) in (\"\")"=w153) -> ("States Out"=w152:string)  [unwired: 14 in]
      }
      frame "UI: Initialize" {
        n89 = local read "Cycle Count Path"() -> (w155:path)
        n90 = Unbundle By Name(w175) -> ("Label Com Array"=w164:string[][])
        n91 = call <vilib>:"Check if File or Folder Exists.vi"("path"=w155) -> ("file or folder exists?"=w154:bool)  [unwired: 8 in, 2 out]
        n92 = Transpose 2D Array(2D array=w164) -> (transposed array=w165:string[][])
        n93 = case shown="True" w154 {
          tunnel: [dbl[][] [[0.0, 0.0], [0.0, 0.0], [0.0, 0.0], [0.0, 0.0]] ("all rows") w182] -> w160
          tunnel: w155 -> [_ w180]
          frame False {
          }
          frame True {
            n94 = call-poly <vilib>:"Read From Spreadsheet File.vi"("delimiter (\\t)"="," ("element"), "file path (dialog if empty)"=w180) -> ("all rows"=w182:dbl[][])  [unwired: 5 in, 4 out]
          }
        }
        n95 = call "UTILITY Array Get 1D Row From 2D String.vi"("all rows"=w165, "row index"=0) -> ("row"=w162:string[])  [unwired: 13 in]
        n96 = Index Array(array=w160, index (col)=1 ("disabled index (col)")) -> (element=w158:dbl[])  [unwired: 1 in]
        n97 = property on="Select Station" class="CmbBox"("Strings[]"=w162) -> ()  [unwired: 2 in, 2 out]
        n98 = Delete From Array(array=w158, length=4) -> (deleted portion=w156:dbl[])  [unwired: 1 in, 1 out]
        n99 = for {
          tunnel: w164 -> [w197] mode=indexing
          tunnel: [w186] -> w173 mode=indexing
          tunnel: [w191] -> w167 mode=indexing
          tunnel: [w189] -> w172
          tunnel: [w185] -> w161 mode=indexing
          tunnel: w156 -> [w183] mode=indexing
          i -> [w190]
          n100 = Index Array(array=w197, index #1=0 ("index"), index #2=1 ("index")) -> (element #1=w193:string, element #2=w192:string)
          n101 = Decimal String To Number(string=w192) -> (number=w188:i32)  [unwired: 2 in, 1 out]
          n102 = To Unsigned Long Integer(number=w183) -> (unsigned 32bit integer=w184:u32)
          n103 = Bundle By Name(cluster=T4 {"Label"="M1", "Color"=0, "Last Read Status"=enum."Err", "Command:Data"="", "Err Count"=0, "Cycle Count"=0} ("Location:IND,Status,Message,No Com Count, Cycle Count"), "Label"=w193, "Cycle Count"=w184) -> (w191:T4)
          n104 = To Unsigned Byte Integer(number=w188) -> (unsigned 8bit integer=w186:u8)
          n105 = Increment(x=w190) -> (x+1=w189:i32)
          n106 = Bundle By Name(cluster=T2 {"Color"=0, "Last Read Status"=enum."Err", "Command:Data"="", "Com Port"=0, "Time(S)"=0.0, "Err Count"=0} ("Dryer Status Serial Data In"), "Com Port"=w186) -> (w185:T2)
        }
        n107 = call <vilib>:"Add State(s) to Queue__jki_lib_state_machine.vi"("State(s) in (\"\")"=w178) -> ("States Out"=w177:string)  [unwired: 14 in]
        n108 = local write "UI Array"(w167) -> ()
        n109 = Bundle By Name(cluster=w175, "UI Array"=w167, "Com Array"=w173) -> (w174:T7)
        n110 = local write "Status Array Out"(w161) -> ()
        n111 = In Range and Coerce(upper limit=20, x=w172, lower limit=1) -> (coerced(x)=w169:i32, In Range?=w168:bool)
        n112 = Not(x=w168) -> (.not. x?=w166:bool)
        n113 = property on="UI Array" class="Arr (strict)"("Number of Rows"=w169, "VertScroll"=w166) -> ()  [unwired: 2 in, 2 out]
      }
      frame "Init Com Ports" {
        n114 = Unbundle By Name(w204) -> ("Com Array"=w203:u8[])
        n115 = for {
          tunnel: w203 -> [w214] mode=indexing
          shift-right: [w212] -> w201
          shift-left: w202 -> [w212]
          tunnel: [w213] -> w200
          stop <- w212 stop-if-true
          # "Send Command (Enable Debug)"
          n116 = call "UTILITY Com Chan Type Conversion.vi"("Com Chan"=w214) -> ("VISA resource name"=w213:refnum<visa-resource-name>)  [unwired: 11 in, 3 out]
        }
        n117 = case shown="No Error" w201 {
          tunnel: w200 -> [_ w210]
          tunnel: w199 -> [_ w209]
          tunnel: [_ "Exit" ("State(s) in Front (\"\")")] -> w198
          frame No Error {
          }
          frame Error {
            n118 = call "UTILITY Com Chan Type Conversion.vi"("Com Chan In"=w210) -> ("Com Text 2"=w207:string)  [unwired: 11 in, 3 out]
            n119 = Concatenate Strings(w209, w207) -> (w211:string)
            n120 = One Button Dialog(message=w211) -> ()  [unwired: 1 in, 1 out]
          }
        }
        n121 = call <vilib>:"Add State(s) to Queue__jki_lib_state_machine.vi"("State(s) in Front (\"\")"=w198, "State(s) in (\"\")"=w206) -> ("States Out"=w205:string)  [unwired: 13 in]
      }
      frame "Init Power" {
        w221 = TRUE  # Valves Off
        # "Initialize the User Interface, here.\n(this is called automatically, by the Macro: Init)"
        n122 = Unbundle By Name(w218) -> ("task out"=w217:refnum<k21>, "Power"=w215:bool[])
        n123 = Build Array(w221, w221, w221, w221) -> (w220:bool[])
        n124 = Build Array (concatenate)(w220, w215) -> (w216:bool[])
        n125 = Boolean Array To Number(Boolean array=w216) -> (number=w219:u32)
        n126 = call-poly <vilib>:"DAQmx Write.vi"("task/channels in"=w217, "data"=w219, "error in"=w223) -> ("error out"=w222:errorcluster)  [unwired: 10 in, 2 out]
        n127 = call <vilib>:"Add State(s) to Queue__jki_lib_state_machine.vi"("State(s) in (\"\")"=w225) -> ("States Out"=w224:string)  [unwired: 14 in]
      }
      frame "Init Labels" {
        n128 = Unbundle By Name(w234) -> ("Label Com Array"=w235:string[][])
        n129 = call "WILT Panel SS Station Labels.vi"("Label Com Array"=w235) -> ("Array Out"=w226:string[][])  [unwired: 10 in]
        n130 = Transpose 2D Array(2D array=w226) -> (transposed array=w229:string[][])
        n131 = local read "Config File"() -> (w232:path)
        n132 = call "UTILITY Array Get 1D Row From 2D String.vi"("all rows"=w229, "row index"=0) -> ("row"=w227:string[])  [unwired: 13 in]
        n133 = local write "Label Com Array"(w226) -> ()
        n134 = property on="Select Station" class="CmbBox"("Strings[]"=w227) -> ()  [unwired: 2 in, 2 out]
        n135 = call-poly <vilib>:"Write To Spreadsheet File.vi"("delimiter (\\t)"="," ("delimiter (\\t)"), "2D data"=w226, "file path (dialog if empty)"=w232) -> ()  [unwired: 5 in, 1 out]
        n136 = Bundle By Name(cluster=w234, "Label Com Array"=w226) -> (w233:T7)
        n137 = call <vilib>:"Add State(s) to Queue__jki_lib_state_machine.vi"("State(s) in (\"\")"=w237) -> ("States Out"=w236:string)  [unwired: 14 in]
      }
      frame "Send Restart" {
        # "Send GEA Command"
        # "send the restart command"
        n138 = case shown="\"D\"" w243 {
          tunnel: [2 ("index") 3 ("index") 0 ("index") 1 ("index")] -> w241
          frame "C", Default {
          }
          frame "D" {
          }
          frame "A" {
          }
          frame "B" {
          }
        }
        n139 = Unbundle By Name(w246) -> ("Com Array"=w242:u8[])
        n140 = Index Array(array=w242, index=w241) -> (element=w240:u8)
        n141 = call "UTILITY Com Chan Type Conversion.vi"("Com Chan"=w240) -> ("VISA resource name"=w245:refnum<visa-resource-name>)  [unwired: 11 in, 3 out]
        n142 = case shown="Error" w238 {
          selector: w238 -> [w253 w255]
          tunnel: w245 -> [_ w258]
          tunnel: w244 -> [_ w257]
          tunnel: [w253 w254] -> w239
          frame No Error {
          }
          frame Error {
            n143 = call "UTILITY Counter.vi"() -> ("Count"=→"Restart Err Count":dbl)  [unwired: 11 in]
            n144 = call "UTILITY Com Chan Type Conversion.vi"("Com Chan In"=w258) -> ("Com Text"=w259:string)  [unwired: 11 in, 3 out]
            n145 = Concatenate Strings(w257, w259) -> (→"Com Er Mess":string)
            n146 = call <vilib>:"Clear Errors.vi"("error in (no error)"=w255) -> ("error out"=w254:errorcluster)  [unwired: 5 in, 1 out]
          }
        }
        n147 = call <vilib>:"Add State(s) to Queue__jki_lib_state_machine.vi"("State(s) in (\"\")"=w248) -> ("States Out"=w247:string)  [unwired: 14 in]
      }
      frame "UI: Cursor Set" {
        # "Argument"
        # "Set and Unset Cursor Busy.\n(Usage: \"UI: Cursor Set >> Busy|Idle\")"
        n148 = case shown="\"Idle\", Default" w261 {
          tunnel: w263 -> [w268 w270]
          tunnel: [w267 w269] -> w262
          frame "Idle", Default {
            n149 = call <vilib>:"Unset Busy.vi"("error in (no error)"=w268) -> ("error out"=w267:errorcluster)  [unwired: 10 in]
          }
          frame "Busy" {
            n150 = call <vilib>:"Set Busy.vi"("error in (no error)"=w270) -> ("error out"=w269:errorcluster)  [unwired: 9 in, 1 out]
          }
        }
        n151 = call <vilib>:"Add State(s) to Queue__jki_lib_state_machine.vi"("State(s) in (\"\")"=w266) -> ("States Out"=w265:string)  [unwired: 14 in]
      }
      frame "UI: Front Panel State" {
        # "Argument"
        # "Set Front Panel Open or Closed\n(Usage: \"UI: Front Panel State >> Open|Close\")"
        n152 = Unbundle By Name(w273) -> ("Core.Current VI Reference"=w272:refnum<vi>)
        n153 = case shown="\"Open\", Default" w271 {
          tunnel: w275 -> [w281 w294]
          tunnel: [w283 w295] -> w274
          tunnel: w272 -> [w282 w292]
          frame "Open", Default {
            n154 = property class="VI"(reference=w282, error in=w281) -> (reference out=w279:refnum<vi>, error out=w280:errorcluster, "Front Panel.Open"=w278:bool)
            n155 = case shown="False" w278 {
              tunnel: [w286 w289] -> w283
              tunnel: w280 -> [w285 w289]
              tunnel: w279 -> [w284 _]
              frame False {
                n156 = invoke class="VI" method="FP.Open"(reference=w284, error in=w285, "Activate"=TRUE, "State"=T6."Standard") -> (error out=w286:errorcluster)  [unwired: 1 in, 4 out]
              }
              frame True {
              }
            }
          }
          frame "Close" {
            n157 = property class="VI"(reference=w292, error in=w294) -> (reference out=w291:refnum<vi>, error out=w293:errorcluster, "Front Panel.Open"=w290:bool)
            n158 = case shown="True" w290 {
              tunnel: [w296 w299] -> w295
              tunnel: w293 -> [w296 w298]
              tunnel: w291 -> [_ w297]
              frame False {
              }
              frame True {
                n159 = invoke class="VI" method="FP.Close"(reference=w297, error in=w298) -> (error out=w299:errorcluster)  [unwired: 1 in, 2 out]
              }
            }
          }
        }
        n160 = call <vilib>:"Add State(s) to Queue__jki_lib_state_machine.vi"("State(s) in (\"\")"=w277) -> ("States Out"=w276:string)  [unwired: 14 in]
      }
      frame "---------- Macro ----------" {
        # "Do not put any code in this frame.\n(It is a separator no-op. You can make a copy of this frame to create a new Macro frame)"
        n161 = call <vilib>:"Add State(s) to Queue__jki_lib_state_machine.vi"("State(s) in (\"\")"=w303) -> ("States Out"=w302:string)  [unwired: 14 in]
      }
      frame "Macro: Initialize" {
        w304 = "Data: Initialize\nInitialize Core Data\nUI: Initialize\nUI: Front Panel State >> Open\nInit Com Ports"  # Data: Initialize Initialize Core Data UI: Initialize UI: Front Panel State >> Open Init Com Ports
        # "Initialization Macro\n(This is called once, when the VI starts)"
        n162 = call <vilib>:"Add State(s) to Queue__jki_lib_state_machine.vi"("State(s) in Front (\"\")"=w304, "State(s) in (\"\")"=w308) -> ("States Out"=w307:string)  [unwired: 13 in]
      }
      frame "Macro: Exit" {
        # "Exit Macro\n(This is called once, when the VI exits)"
        n163 = Unbundle By Name(w315) -> ("Core.Close Panel on Exit?"=w314:bool)
        n164 = Select(t="UI: Front Panel State >> Close", s=w314, f="") -> (s? t:f=w311:string)
        n165 = call <vilib>:"Add State(s) to Queue__jki_lib_state_machine.vi"("State(s) in (\"\")"=w311, "State(s) at Back (\"\")"="Data: Cleanup\nExit") -> ("States Out"=w309:string)  [unwired: 13 in]
        n166 = call <vilib>:"Add State(s) to Queue__jki_lib_state_machine.vi"("State(s) in Front (\"\")"=w309, "State(s) in (\"\")"=w318) -> ("States Out"=w317:string)  [unwired: 13 in]
      }
      frame "---------- New Category ----------" {
        # "Template Separator\n(You can make a copy of, or modify, this frame)"
        n167 = call <vilib>:"Add State(s) to Queue__jki_lib_state_machine.vi"("State(s) in (\"\")"=w322) -> ("States Out"=w321:string)  [unwired: 14 in]
      }
      frame "Get Currents" {
        n168 = Unbundle By Name(w342) -> ("UI Array"=w343:T4[])
        n169 = call "WILT Rising Edge Latch.vi"() -> ("Rising Edge Out"=w326:bool[])  [unwired: 11 in]
        "Rising Edge Out" <- w326
        n170 = local read "Max Len"() -> (w323:i32)
        n171 = stacked-sequence {
          tunnel: "Up Lim" -> [w377 w392 w407 w422]
          tunnel: "Low Lim" -> [w376 w391 w406 w421]
          tunnel: w323 -> [w373 w388 w404 w418]
          tunnel: [w369 _ _ _] -> w334
          tunnel: [_ w385 _ _] -> w333
          tunnel: [_ _ w401 _] -> w332
          tunnel: [_ _ _ w417] -> w338
          tunnel: "Low Lim 2" -> [w372 w387 w402 w416]
          frame #0 {
            n172 = call "WILT SS Current Test.vi"("Lower Limit 2"=w372, "Lower Limit"=w376, "Y 2"="A Data 2", "Y"="A Data", "Upper Limit"=w377) -> ("Out of Bounds"=w370:bool, "Waveform Chart"=→"Station A: L1 Current":waveform(dbl)[])  [unwired: 5 in]
            "A Alarm" <- w370
            n173 = Array Size(array="A Data") -> (size(s)=w374:i32)
            n174 = Equal?(x=w374, y=w373) -> (x = y?=w371:bool)
            n175 = case shown="True" w371 {
              tunnel: [_ w381] -> w369
              tunnel: w370 -> [_ w380]
              frame False {
              }
              frame True {
                n176 = case shown="False" w380 {
                  tunnel: ["Write >> A" "Send Restart >> A"] -> w381
                  frame True {
                  }
                  frame False {
                  }
                }
              }
            }
          }
          frame #1 {
            n177 = call "WILT SS Current Test.vi"("Lower Limit 2"=w387, "Lower Limit"=w391, "Y 2"="B Data 2", "Y"="B Data", "Upper Limit"=w392) -> ("Out of Bounds"=w384:bool, "Waveform Chart"=→"Station B: L1 Current":waveform(dbl)[])  [unwired: 5 in]
            "B Alarm" <- w384
            n178 = Array Size(array="B Data") -> (size(s)=w389:i32)
            n179 = Equal?(x=w388, y=w389) -> (x = y?=w386:bool)
            n180 = case shown="True" w386 {
              tunnel: [_ w396] -> w385
              tunnel: w384 -> [_ w395]
              frame False {
              }
              frame True {
                n181 = case shown="True" w395 {
                  tunnel: ["Write >> B" "Send Restart >> B"] -> w396
                  frame True {
                  }
                  frame False {
                  }
                }
              }
            }
          }
          frame #2 {
            n182 = call "WILT SS Current Test.vi"("Lower Limit 2"=w402, "Lower Limit"=w406, "Y 2"="C Data 2", "Y"="C Data", "Upper Limit"=w407) -> ("Out of Bounds"=w399:bool, "Waveform Chart"=→"Station C: L1 Current":waveform(dbl)[])  [unwired: 5 in]
            "C Alarm" <- w399
            n183 = Array Size(array="C Data") -> (size(s)=w405:i32)
            n184 = Equal?(x=w404, y=w405) -> (x = y?=w400:bool)
            n185 = case shown="True" w400 {
              tunnel: [_ w411] -> w401
              tunnel: w399 -> [_ w410]
              frame False {
              }
              frame True {
                n186 = case shown="False" w410 {
                  tunnel: ["Write >> C" "Send Restart >> C"] -> w411
                  frame True {
                  }
                  frame False {
                  }
                }
              }
            }
          }
          frame #3 {
            n187 = call "WILT SS Current Test.vi"("Lower Limit 2"=w416, "Lower Limit"=w421, "Y 2"="D Data 2", "Y"="D Data", "Upper Limit"=w422) -> ("Out of Bounds"=w414:bool, "Waveform Chart"=→"Station D: L1 Current":waveform(dbl)[])  [unwired: 5 in]
            "D Alarm" <- w414
            n188 = Array Size(array="D Data") -> (size(s)=w420:i32)
            n189 = Equal?(x=w418, y=w420) -> (x = y?=w415:bool)
            n190 = case shown="True" w415 {
              tunnel: [_ w426] -> w417
              tunnel: w414 -> [_ w425]
              frame False {
              }
              frame True {
                n191 = case shown="True" w425 {
                  tunnel: ["Write >> D" "Send Restart >> D"] -> w426
                  frame True {
                  }
                  frame False {
                  }
                }
              }
            }
          }
        }
        n192 = for {
          tunnel: w326 -> [w368] mode=indexing
          tunnel: w343 -> [w367] mode=indexing
          tunnel: [w364] -> w329 mode=indexing
          tunnel: [TRUE] -> w344
          tunnel: [w360] -> w327 mode=indexing
          tunnel: [w356] -> w328 mode=indexing
          n193 = Boolean To (0,1)(Boolean=w368) -> (0, 1=w365:i16)
          n194 = Unbundle By Name(w367) -> ("Label"=w357:string, "Cycle Count"=w366:u32)
          n195 = To Unsigned Long Integer(number=w365) -> (unsigned 32bit integer=w355:u32)
          n196 = Add(x=w366, y=w355) -> (x+y=w359:u32)
          n197 = Quotient & Remainder(x=w359, y="Cycle Save Multiple") -> (x-y*floor(x/y)=w361:u32)  [unwired: 1 out]
          n198 = Bundle By Name(cluster=w367, "Cycle Count"=w359) -> (w364:T4)
          n199 = Equal To 0?(x=w361) -> (x = 0?=w360:bool)
          n200 = Number To Decimal String(number=w359) -> (decimal integer string=w358:string)  [unwired: 1 in]
          n201 = Build Array(w357, w358) -> (w356:string[])
        }
        n202 = And(x=w327, y=w326) -> (x .and. y?=w325:bool[])
        n203 = call "WILT Rising Edge Latch.vi"("Reset"=w344) -> ()  [unwired: 10 in, 1 out]
        n204 = call <vilib>:"Add State(s) to Queue__jki_lib_state_machine.vi"("State(s) in Front (\"\")"=w334, "State(s) in (\"\")"=w335) -> ("States Out"=w336:string)  [unwired: 13 in]
        n205 = Or Array Elements(Boolean array=w325) -> (logical OR=w324:bool)
        n206 = local write "UI Array"(w329) -> ()
        n207 = case shown="True" w324 {
          tunnel: w328 -> [_ w350]
          frame False {
          }
          frame True {
            n208 = call "UTILITY Log String to Spreadsheet.vi"("String"="Count Log", "FileName"="Cycle Count Path") -> ("error out"=w347:errorcluster)  [unwired: 9 in]
            n209 = flat-sequence {
              tunnel: w350 -> [w354]
              tunnel: "Cycle Count Path" -> [w352]
              tunnel: w347 -> [_]
              frame #0 {
                n210 = call-poly <vilib>:"Write To Spreadsheet File.vi"("delimiter (\\t)"="," ("delimiter (\\t)"), "append to file? (new file:F)"=TRUE, "2D data"=w354, "file path (dialog if empty)"=w352) -> ()  [unwired: 4 in, 1 out]
              }
            }
          }
        }
        n211 = call <vilib>:"Add State(s) to Queue__jki_lib_state_machine.vi"("State(s) in Front (\"\")"=w333, "State(s) in (\"\")"=w336) -> ("States Out"=w337:string)  [unwired: 13 in]
        n212 = call <vilib>:"Add State(s) to Queue__jki_lib_state_machine.vi"("State(s) in Front (\"\")"=w332, "State(s) in (\"\")"=w337) -> ("States Out"=w331:string)  [unwired: 13 in]
        n213 = Bundle By Name(cluster=w342, "UI Array"=w329) -> (w341:T7)
        n214 = call <vilib>:"Add State(s) to Queue__jki_lib_state_machine.vi"("State(s) in Front (\"\")"=w338, "State(s) in (\"\")"=w331) -> ("States Out"=w346:string)  [unwired: 13 in]
      }
      frame "Check Power" {
        # "Last read current."
        # "True means turn power off."
        n215 = global read "Globals SS.vi" "D L1 index"() -> (w430:i32)
        n216 = global read "Globals SS.vi" "C L1 index"() -> (w431:i32)
        n217 = global read "Globals SS.vi" "B L1 index"() -> (w432:i32)
        n218 = global read "Globals SS.vi" "A L1 Index"() -> (w433:i32)
        n219 = local read "Max Len"() -> (w429:i32)
        n220 = local read "D Data"() -> (w441:dbl[])
        n221 = local read "A Data"() -> (w448:dbl[])
        n222 = local read "B Data"() -> (w444:dbl[])
        n223 = local read "C Data"() -> (w443:dbl[])
        n224 = Array Size(array=w441) -> (size(s)=w442:i32)
        n225 = Array Size(array=w448) -> (size(s)=w447:i32)
        n226 = Array Size(array=w444) -> (size(s)=w445:i32)
        n227 = Array Size(array=w443) -> (size(s)=w440:i32)
        n228 = local read "Currents"() -> (w468:dbl[])
        n229 = local read "B Alarm"() -> (w454:bool)
        n230 = local read "A Alarm"() -> (w453:bool)
        n231 = local read "C Alarm"() -> (w455:bool)
        n232 = local read "D Alarm"() -> (w456:bool)
        n233 = Greater Or Equal?(x=w440, y=w429) -> (x >= y?=w437:bool)
        n234 = Greater Or Equal?(x=w442, y=w429) -> (x >= y?=w436:bool)
        n235 = Greater Or Equal?(x=w447, y=w429) -> (x >= y?=w439:bool)
        n236 = Greater Or Equal?(x=w445, y=w429) -> (x >= y?=w438:bool)
        n237 = Index Array(array=w468, index #1=w433, index #2=w432, index #3=w431, index #4=w430) -> (element #1=w467:dbl, element #2=w466:dbl, element #3=w465:dbl, element #4=w464:dbl)
        n238 = local read "Off On Threshold"() -> (w434:dbl)
        n239 = Bundle(w439, w438, w437, w436) -> (w446:cluster{bool, bool, bool, bool})  [unwired: 1 in]
        n240 = Bundle("A Alarm"=w453, "B Alarm"=w454, "C Alarm"=w455, "D Alarm"=w456) -> (w452:T9)  [unwired: 1 in]
        n241 = Bundle("Waveform"=w467, "Waveform"=w466, "Waveform"=w465, "Waveform"=w464) -> (w463:T10)  [unwired: 1 in]
        n242 = Cluster To Array(cluster=w446) -> (array=w435:bool[])
        n243 = Cluster To Array(cluster=w463) -> (array=w462:dbl[])
        n244 = Cluster To Array(cluster=w452) -> (array=w451:bool[])
        n245 = Greater?(x=w462, y=w434) -> (0:w450:bool[])
        n246 = Compound Arithmetic op=AND(w451, w450, w435) -> (w449:bool[])
        n247 = Not(x=w449) -> (.not. x?=w461:bool[])
        n248 = Or Array Elements(Boolean array=w461) -> (logical OR=w458:bool)
        n249 = case shown="True" w458 {
          tunnel: [_ "Init Power" ("State(s) in Front (\"\")")] -> w457
          frame False {
          }
          frame True {
          }
        }
        n250 = Bundle By Name(cluster=w470, "Power"=w449) -> (w469:T7)
        n251 = call <vilib>:"Add State(s) to Queue__jki_lib_state_machine.vi"("State(s) in Front (\"\")"=w457, "State(s) in (\"\")"=w459) -> ("States Out"=w460:string)  [unwired: 13 in]
      }
      frame "Read" {
        # "read all the com array ports, and update the gui"
        n252 = call "UTILITY Counter.vi"() -> ("Count"=→"Read Serial Count":dbl)  [unwired: 11 in]
        n253 = flat-sequence {
          tunnel: [w482] -> _
          frame #0 {
            n254 = local read "Status Array Out"() -> (w482:T2[])
            n255 = local write "Reading"(TRUE ("Reading")) -> ()
          }
        }
        n256 = Unbundle By Name(w477) -> ("Label Com Array"=w475:string[][], "UI Array"=w478:T4[])  [unwired: 1 out]
        n257 = for {
          tunnel: w478 -> [w497] mode=indexing
          tunnel: [w493] -> w474 mode=indexing
          tunnel: w475 -> [w492] mode=indexing
          i -> [w489]
          n258 = Index Array(array=w492, index=0) -> (element=w488:string)
          n259 = Unbundle By Name() -> ("Color"=w496:u32, "Last Read Status"=w495:T3, "Command:Data"=w494:string, "Err Count"=w490:u32)  [unwired: 1 in]
          n260 = case shown="True" {
            selector: _ -> [_ _]
            tunnel: w488 -> [_ w512]
            tunnel: [_ w510] -> w487
            frame False {
            }
            frame True {
              n261 = Concatenate Strings(w512, "," ("string")) -> (w510:string)  [unwired: 1 in]
            }
          }
          n262 = case shown="0, Default" w489 {
            tunnel: w487 -> [w498 w501 w504 w507]
            frame 0, Default {
              n263 = local read "A Array"() -> (w499:string[][])
              n264 = call "WILT Array Insert on Bottom.vi"("New String"=w498, "appended array"=w499) -> ("output array"=→"A Array":string[][])  [unwired: 9 in]
            }
            frame 1 {
              n265 = local read "B Array"() -> (w502:string[][])
              n266 = call "WILT Array Insert on Bottom.vi"("New String"=w501, "appended array"=w502) -> ("output array"=→"B Array":string[][])  [unwired: 9 in]
            }
            frame 2 {
              n267 = local read "C Array"() -> (w505:string[][])
              n268 = call "WILT Array Insert on Bottom.vi"("New String"=w504, "appended array"=w505) -> ("output array"=→"C Array":string[][])  [unwired: 9 in]
            }
            frame 3 {
              n269 = local read "D Array"() -> (w508:string[][])
              n270 = call "WILT Array Insert on Bottom.vi"("New String"=w507, "appended array"=w508) -> ("output array"=→"D Array":string[][])  [unwired: 9 in]
            }
          }
          n271 = Bundle By Name(cluster=w497, "Color"=w496, "Last Read Status"=w495, "Command:Data"=w494, "Err Count"=w490) -> (w493:T4)
        }
        n272 = Bundle By Name(cluster=w477, "UI Array"=w474) -> (w476:T7)
        n273 = flat-sequence {
          tunnel: w474 -> [w486]
          frame #0 {
            n274 = local write "UI Array"(w486) -> ()
            "Reading" <- FALSE ("Reading")
            "Ready" <- TRUE ("Reading")
          }
        }
        n275 = call <vilib>:"Add State(s) to Queue__jki_lib_state_machine.vi"("State(s) in (\"\")"=w481) -> ("States Out"=w480:string)  [unwired: 14 in]
      }
      frame "Write" {
        w514 = "_" ("string")
        # "SS"
        # "Writes the data file."
        n276 = Unbundle By Name(w542) -> ("Save File Path"=w518:path, "Label Com Array"=w528:string[][], "Last Hour"=w536:string, "Computer Name"=w529:string)
        n277 = case shown="\"A\", Default" w513 {
          tunnel: w528 -> [w553 w561 w569 w577]
          tunnel: [w550 w558 w566 w574] -> w527
          tunnel: [w549 w557 w565 w573] -> w526
          tunnel: ["A save" "B save" "C save" "D save"] -> w525
          tunnel: [w547 w555 w563 w571] -> w520
          tunnel: [w546 w554 w562 w570] -> w523
          frame "A", Default {
            n278 = local read "A Data"() -> (w547:dbl[])
            n279 = local read "A Data 2"() -> (w546:dbl[])
            n280 = local read "A Array"() -> (w549:string[][])
            n281 = Index Array(array=w553, index (row)=0, index (col)=0 ("disabled index (col)")) -> (element=w550:string)
          }
          frame "B" {
            n282 = local read "B Data"() -> (w555:dbl[])
            n283 = local read "B Data 2"() -> (w554:dbl[])
            n284 = local read "B Array"() -> (w557:string[][])
            n285 = Index Array(array=w561, index (row)=1, index (col)=0 ("disabled index (col)")) -> (element=w558:string)
          }
          frame "C" {
            n286 = local read "C Data"() -> (w563:dbl[])
            n287 = local read "C Data 2"() -> (w562:dbl[])
            n288 = local read "C Array"() -> (w565:string[][])
            n289 = Index Array(array=w569, index (row)=2, index (col)=0 ("disabled index (col)")) -> (element=w566:string)
          }
          frame "D" {
            n290 = local read "D Data"() -> (w571:dbl[])
            n291 = local read "D Data 2"() -> (w570:dbl[])
            n292 = local read "D Array"() -> (w573:string[][])
            n293 = Index Array(array=w577, index (row)=3, index (col)=0 ("disabled index (col)")) -> (element=w574:string)
          }
        }
        n294 = Format Date/Time String(time format string (%c)="%H") -> (date/time string=w537:string)  [unwired: 2 out]
        n295 = Equal?(x=w536, y=w537) -> (x = y?=w533:bool)
        n296 = Equal?(x=w536, y="Backup Hour") -> (x = y?=w532:bool)
        n297 = Not Equal?(x=w520, y=w525) -> (x != y?=w524:bool)
        n298 = Build Array(w520, w523) -> (w522:dbl[][])
        n299 = Format Date/Time String(time format string (%c)="%Y%m%d_%H%M%S_") -> (date/time string=w531:string)  [unwired: 2 out]
        n300 = Not(x=w533) -> (.not. x?=w534:bool)
        n301 = Transpose 2D Array(2D array=w522) -> (transposed array=w521:dbl[][])
        n302 = And(x=w534, y=w532) -> (x .and. y?=w530:bool)
        "robo?" <- w530
        n303 = Concatenate Strings(w531, w529, w514, w527, w514, w513, "_SS_Data.csv" ("string")) -> (w517:string)
        n304 = call "WILT Filename Generate SS.vi"("name or relative path"=w517, "path"=w518) -> ("appended path"=w516:path)  [unwired: 8 in, 1 out]
        n305 = case shown="True" w530 {
          frame False {
          }
          frame True {
            n306 = call <vilib>:"System Exec.vi"("command line"="\"C:\\Program Files\\GE\\Start Stop\\robocopy_backup.bat\"" ("data backup command line")) -> ("error out"=→"Saving":errorcluster)  [unwired: 7 in, 3 out]
          }
        }
        n307 = case shown="True" w524 {
          tunnel: w516 -> [w578 w585]
          tunnel: [w578 w579] -> w539
          tunnel: w526 -> [_ w592]
          tunnel: w521 -> [_ w590]
          tunnel: w513 -> [_ w587]
          tunnel: w520 -> [_ w586]
          tunnel: string[] ["L1 Array, L2 Array(Amps) in 0.5 sec samples, then Com Traffic preceding failure "] ("1D data") -> [_ w583]
          frame False {
          }
          frame True {
            w582 = TRUE ("transpose? (no:F)")
            w589 = "," ("delimiter (\\t)")
            n308 = call-poly <vilib>:"Write To Spreadsheet File.vi"("1D data"=w583, "file path (dialog if empty)"=w585) -> ("new file path (Not A Path if cancelled)"=w584:path)  [unwired: 6 in]
            n309 = case shown="\"D\"" w587 {
              tunnel: w586 -> [w593 w594 w595 w596]
              frame "A", Default {
                n310 = local write "A save"(w593) -> ()
              }
              frame "B" {
                n311 = local write "B save"(w594) -> ()
              }
              frame "C" {
                n312 = local write "C save"(w595) -> ()
              }
              frame "D" {
                n313 = local write "D save"(w596) -> ()
              }
            }
            n314 = call-poly <vilib>:"Write To Spreadsheet File.vi"("delimiter (\\t)"=w589, "transpose? (no:F)"=w582, "append to file? (new file:F)"=w582, "2D data"=w590, "file path (dialog if empty)"=w584) -> ("new file path (Not A Path if cancelled)"=w588:path)  [unwired: 3 in]
            n315 = call-poly <vilib>:"Write To Spreadsheet File.vi"("delimiter (\\t)"=w589, "append to file? (new file:F)"=TRUE, "2D data"=w592, "file path (dialog if empty)"=w588) -> ("new file path (Not A Path if cancelled)"=w580:path)  [unwired: 4 in]
            n316 = Set Permissions(7:i16 0 ("permissions"), 11:w580) -> (3:w579:path)  [unwired: 3 in, 1 out]
          }
        }
        "Current Filename" <- w539
        n317 = Bundle By Name(cluster=w542, "Last Hour"=w537) -> (w541:T7)
        n318 = call <vilib>:"Add State(s) to Queue__jki_lib_state_machine.vi"("State(s) in (\"\")"=w545) -> ("States Out"=w544:string)  [unwired: 14 in]
      }
      frame "Add Select Data" {
        # "Your code here.\n(You can make a copy of, or modify, this frame)"
        n319 = Unbundle By Name(w613) -> ("Label Com Array"=w612:string[][], "UI Array"=w611:T4[])
        n320 = for {
          tunnel: w612 -> [w634] mode=indexing
          tunnel: w611 -> [w629] mode=indexing
          tunnel: [w628] -> w610
          tunnel: [w628] -> w608
          stop <- w630 stop-if-true
          n321 = Unbundle By Name(w629) -> ("Command:Data"=w628:string)
          n322 = Index Array(array=w634, index=0) -> (element=w631:string)
          n323 = Equal?(x=w631, y="Select Station") -> (x = y?=w630:bool)
        }
        n324 = global read "Globals SS.vi" "Max Length of Display Data"() -> (w605:i32)
        n325 = String Length(string=w608) -> (length=w607:i32)
        n326 = Greater Than 0?(x=w607) -> (x > 0?=w606:bool)
        n327 = case shown="True" w606 {
          tunnel: w610 -> [_ w626]
          tunnel: "Command:Data" -> [w617 w625]
          tunnel: [w617 w627] -> w604
          tunnel: w605 -> [_ w619]
          tunnel: "\n--------------------\n" ("string") -> [_ w621]
          frame False {
          }
          frame True {
            n328 = Concatenate Strings(w625, w621, w626) -> (w624:string)
            n329 = String Length(string=w624) -> (length=w623:i32)
            n330 = Subtract(x=w623, y=w619) -> (x-y=w622:i32)
            n331 = In Range and Coerce(upper limit=w619, x=w622, lower limit=0) -> (coerced(x)=w620:i32)  [unwired: 1 out]
            n332 = String Subset(string=w624, offset (0)=w620, length (rest)=w619) -> (substring=w627:string)
          }
        }
        n333 = Search and Replace String(input string=w604, search string="\n") -> (number of replacements=w602:i32)  [unwired: 6 in, 3 out]
        n334 = local write "Command:Data"(w604) -> ()
        n335 = Subtract(x=w602, y=10) -> (x-y=w600:i32)
        n336 = property on="Command:Data" class="Str"("Text.Scroll Position"=w600) -> ()  [unwired: 2 in, 2 out]
        n337 = call <vilib>:"Add State(s) to Queue__jki_lib_state_machine.vi"("State(s) in (\"\")"=w616) -> ("States Out"=w615:string)  [unwired: 14 in]
      }
    }
  }
  "Stop" <- w3
  n338 = while "Gather SS Data State Machine" {
    shift-right: [w638] -> _
    shift-left: _ -> [w637]
    shift-right: [w641] -> _
    shift-left: _ -> [w635]
    shift-right: [w640] -> _
    shift-left: w1 -> [w642]
    stop <- w639 stop-if-true
    w636 = 500  # Timeout
    n339 = call <vilib>:"Parse State Queue__jki_lib_state_machine.vi"("State Queue"=w642, "Error In (no error)"=w635) -> ("Remaining States"=w644:string, "Current State"=w645:string, "Arguments"=w643:string)  [unwired: 11 in]
    n340 = case shown="\"Check for Rising Edge\"" w645 {
      selector: w645 -> [_ _ w668 _ _ _ _ _ _ _ _ _ _ _ _ _]
      tunnel: w644 -> [w652 w667 w672 w684 w689 w693 w714 w732 w738 w742 w766 w801 w822 w855 w888 w921]
      tunnel: w643 -> [_ _ _ _ _ _ _ _ _ _ _ _ _ _ _ _]
      tunnel: w637 -> [w650 w664 w670 w681 w687 w690 _ w718 w736 w739 w763 w798 w819 w852 w885 w918]
      tunnel: [w649 w665 w674 errorcluster {"status"=FALSE, "code"=0, "source"=""} ("error out") w686 w691 w706 w724 w733 w740 w758 w799 w820 w853 w886 w919] -> w641
      tunnel: w635 -> [w648 w665 w673 w680 w686 w691 w706 w725 w735 w740 w759 w799 w820 w853 w886 w919]
      tunnel: [w651 w666 w671 w683 w688 w692 w713 w731 w737 w741 w765 w800 w821 w854 w887 w920] -> w640
      tunnel: [_ _ _ _ TRUE _ _ _ _ _ _ _ _ _ _ _] -> w639
      tunnel: [w647 w664 w670 w681 w687 w690 w712 w717 w736 w739 w762 w797 w818 w851 w884 w917] -> w638
      tunnel: w636 -> [w646 _ _ _ _ _ _ _ _ _ _ _ _ _ _ _]
      frame "", "Idle" {
        # "executes when the state queue is empty"
        n341 = event shown="[0] Timeout" {
          selector: _ -> [_]
          dyn-events: _ -> [_]
          timeout: w646 -> [_]
          tunnel: w652 -> [w658]
          tunnel: [w657] -> w651
          tunnel: w650 -> [w655]
          tunnel: [w656] -> w649
          tunnel: w648 -> [w656]
          tunnel: [w655] -> w647
          event Timeout {
            n342 = event-data() -> ()  [unwired: 1 in, 1 out]
            n343 = case shown="True" "Change Lint" {
              tunnel: [w660 "" ("State(s) in Front (\"\")")] -> w654
              frame False {
                n344 = local read "Stop"() -> (w659:bool)
                n345 = case shown="False" w659 {
                  tunnel: ["Read Currents\nCheck for Rising Edge\nAdd Data:A\nAdd Data:B\nAdd Data:C\nAdd Data:D\n" ("State(s) in Front (\"\")") "Data: Cleanup\nExit" ("State(s) in Front (\"\")")] -> w660
                  frame False {
                  }
                  frame True {
                  }
                }
              }
              frame True {
              }
            }
            n346 = call <vilib>:"Add State(s) to Queue__jki_lib_state_machine.vi"("State(s) in Front (\"\")"=w654, "State(s) in (\"\")"=w658) -> ("States Out"=w657:string)  [unwired: 13 in]
          }
        }
      }
      frame "---------- Core ----------" {
        # "Do not put any code in this frame.\n(it is a separator no-op)"
        n347 = call <vilib>:"Add State(s) to Queue__jki_lib_state_machine.vi"("State(s) in (\"\")"=w667) -> ("States Out"=w666:string)  [unwired: 14 in]
      }
      frame Default {
        w677 = 42 items=["No error", "Argument error", "Memory is full", "Out of zone", "End of file", "File already open", "Generic file I/O error", "File not found", "File permission error", "Disk is full", "Duplicate path", "Too many files open", "System feature not enabled", "Resource file not found", "Cannot add resource", "Resource not found", "Image not found", "Image memory error", "Pen does not exist", "Config type invalid", "Config token not found", "Config parse error", "Config memory error", "Bad external code format", "Bad external code offset", "External code not present", "Null window", "Destroy window error", "Null menu", "Print aborted", "Bad print record", "Print driver error", "Windows error during printing", "Memory error during printing", "Print dialog error", "Generic print error", "Invalid device refnum", "Device not found", "Device parameter error", "Device unit error", "Cannot open device", "Device call aborted", "Generic error", "Cancelled by user", "Object ID too low", "Object ID too high", "Object not in heap", "Unknown heap", "Unknown object (invalid DefProc)", "Unknown object (DefProc not in table)", "Message out of range", "Invalid (null) method", "Unknown message", "Manager call not supported", "Bad address", "Network operation in progress", "Network operation timed out", "Connection is busy", "Network attribute not supported", "Network error", "Address in use", "System out of memory", "Connection aborted", "Connection refused", "Not connected", "Already connected", "Connection closed", "Initialization error (interapplication manager)", "Bad occurrence", "Wait on unbound occurrence handler", "Occurrence queue overflow", "Datalog type conflict", "Unused", "Unrecognized type (interapplication manager)", "Memory corrupt", "Failed to make temporary DLL", "Old CIN version", "Drag socket not found", "Failed to load drop-object", "Failed to register OLE object", "Failed to release OLE object", "Format specifier type mismatch", "Unknown format specifier", "Too few format specifiers", "Too many format specifiers", "Scan failed", "Newer CIN version", "Error converting to variant", "Runtime menu error", "Password tampered", "Variant attribute not found", "Incompatible variant data type", "Event data is not available", "Event Store is not present", "Occurrence is not found", "Event Queue is not created", "Event info is not available", "Refnum passed is NULL", "Error retrieving Class GUID", "Error retrieving CoClass GUID", "Error retrieving TypeLib GUID.", "Bad built application magic bytes.", "Specific driver is different from the specific driver associated with the Logical Name.", "There is no session opened to the class driver.", "Max Error", "MAX - Error with config objects", "MAX - Error loading configuration", "MAX - Group not supported"]
        # "Current State"
        # "Do not delete, rename, or modify this frame.\n(this is used to capture unhandled states and typos)"
        # "Handle mistyped state name (developer tool)"
        n348 = Format Into String(format string="Software Exception: Unhandled State \"%s\"." ("message"), error in=w673, w668) -> (resulting string=w676:string, error out=w675:errorcluster)  [unwired: 1 in]
        n349 = call <vilib>:"Error Cluster From Error Code.vi"("show call chain? (False)"=TRUE, "error in (no error)"=w675, "error message (\"\")"=w676, "error code (0)"=w677) -> ("error out"=w674:errorcluster)  [unwired: 5 in]
        n350 = call <vilib>:"Add State(s) to Queue__jki_lib_state_machine.vi"("State(s) in (\"\")"=w672) -> ("States Out"=w671:string)  [unwired: 14 in]
      }
      frame "Error Handler" {
        # "Unhandled Error -- Display it"
        # "Handle any errors here.\nYou can also output any states to clean-up after errors occur"
        # "Clear error"
        n351 = call <vilib>:"General Error Handler.vi"("error in (no error)"=w680) -> ()  [unwired: 10 in, 5 out]
        n352 = call <vilib>:"Add State(s) to Queue__jki_lib_state_machine.vi"("State(s) in Front (\"\")"="/* Post Error States", "State(s) in (\"\")"=w684) -> ("States Out"=w683:string)  [unwired: 13 in]
      }
      frame "Exit" {
        # "Do not put any code in this frame.\n(No errors that occur here will be handled.)"
        n353 = call <vilib>:"Add State(s) to Queue__jki_lib_state_machine.vi"("State(s) in (\"\")"=w689) -> ("States Out"=w688:string)  [unwired: 14 in]
      }
      frame "---------- Data ----------" {
        # "Do not put any code in this frame.\n(It is a separator no-op. You can make a copy of this frame to create a new Data frame)"
        n354 = call <vilib>:"Add State(s) to Queue__jki_lib_state_machine.vi"("State(s) in (\"\")"=w693) -> ("States Out"=w692:string)  [unwired: 14 in]
      }
      frame "Data: Initialize" {
        w695 = bool[] [FALSE, FALSE, FALSE, FALSE]  # Rise
        w696 = dbl[] []  # Old Data
        w697 = dbl[] []  # Read Data
        w698 = dbl[] []  # D Data2
        w699 = dbl[] []  # D Data
        w700 = dbl[] []  # C Data2
        w701 = dbl[] []  # C Data
        w702 = dbl[] []  # B Data2
        w703 = dbl[] []  # B Data
        w704 = dbl[] []  # A Data2
        w705 = dbl[] []  # A Data
        w708 = FALSE  # Dlatch
        w709 = FALSE  # Clatch
        w710 = FALSE  # Blatch
        w711 = FALSE  # Alatch
        # "Initialize the shift-register data, here.\n(data names are defined by what you wire into the bundle function)"
        n355 = property on="Waveform Chart" class="WFChart (strict)"("History Data"=dbl[] []) -> ()  [unwired: 2 in, 2 out]
        n356 = Bundle("Alatch"=w711, "Blatch"=w710, "Clatch"=w709, "Dlatch"=w708, "AI Task"="AI Task", "A Data"=w705, "A Data2"=w704, "B Data"=w703, "B Data2"=w702, "C Data"=w701, "C Data2"=w700, "D Data"=w699, "D Data2"=w698, "Read Data"=w697, "Old Data"=w696, "Rise"=w695) -> (w712:T11)  [unwired: 1 in]
        n357 = call <vilib>:"Add State(s) to Queue__jki_lib_state_machine.vi"("State(s) in (\"\")"=w714) -> ("States Out"=w713:string)  [unwired: 14 in]
      }
      frame "Init: AI" {
        w716 = 10083 items=["default"=-1, "RSE"=10083, "NRSE"=10078, "Differential"=10106, "Pseudodifferential"=12529] ("input terminal configuration")
        w728 = 10123 items=["Finite Samples"=10178, "Continuous Samples"=10123] ("sample mode")
        # "3."
        # "2."
        # "1."
        n358 = call-poly <vilib>:"DAQmx Create Virtual Channel.vi"("maximum value"="Maximum Value", "minimum value"="Minimum Value", "input terminal configuration"=w716, "physical channels"="AI Channel", "error in"=w725) -> ("task out"=w727:refnum<k21>, "error out"=w726:errorcluster)  [unwired: 9 in]
        n359 = call-poly <vilib>:"DAQmx Timing.vi"("task/channels in"=w727, "sample mode"=w728, "samples per channel"="Samples per Channel", "rate"="Rate", "error in"=w726) -> ("task out"=w729:refnum<k21>, "error out"=w730:errorcluster)  [unwired: 9 in]
        n360 = call <vilib>:"DAQmx Start Task.vi"("task/channels in"=w729, "error in"=w730) -> ("task out"=w719:refnum<k21>, "error out"=w724:errorcluster)  [unwired: 12 in]
        n361 = Bundle By Name(cluster=w718, "AI Task"=w719) -> (w717:T11)
        n362 = call <vilib>:"Add State(s) to Queue__jki_lib_state_machine.vi"("State(s) in (\"\")"=w732) -> ("States Out"=w731:string)  [unwired: 14 in]
      }
      frame "Data: Cleanup" {
        # "Cleanup any data and references, here.\n(this is called automatically, by the Macro: Exit)"
        n363 = Unbundle By Name(w736) -> ("AI Task"=w734:refnum<k21>)
        n364 = call <vilib>:"DAQmx Clear Task.vi"("task in"=w734, "error in"=w735) -> ("error out"=w733:errorcluster)  [unwired: 13 in]
        n365 = call <vilib>:"Add State(s) to Queue__jki_lib_state_machine.vi"("State(s) in (\"\")"=w738) -> ("States Out"=w737:string)  [unwired: 14 in]
      }
      frame "---------- New Category ----------" {
        # "Template Separator\n(You can make a copy of, or modify, this frame)"
        n366 = call <vilib>:"Add State(s) to Queue__jki_lib_state_machine.vi"("State(s) in (\"\")"=w742) -> ("States Out"=w741:string)  [unwired: 14 in]
      }
      frame "Read Currents" {
        w743 = 5.0  # 10V=50A
        n367 = Unbundle By Name(w763) -> ("AI Task"=w764:refnum<k21>)
        n368 = call-poly <vilib>:"DAQmx Read.vi"("task/channels in"=w764, "number of samples per channel"=-1, "error in"=w759) -> ("data"=w755:dbl[][], "error out"=w758:errorcluster)  [unwired: 10 in, 1 out]
        "data" <- w755
        n369 = Array Size(array=w755) -> (size(s)=w748:i32[])
        n370 = Multiply Array Elements(1:w748) -> (0:w747:i32)
        n371 = Equal To 0?(x=w747) -> (x = 0?=w746:bool)
        n372 = Index Array(array=w748, index=1) -> (element=w753:i32)
        n373 = case shown="True" w746 {
          tunnel: [_ "Read Currents" ("State(s) in Front (\"\")")] -> w745
          frame False {
          }
          frame True {
          }
        }
        n374 = Decrement(x=w753) -> (x-1=w749:i32)
        n375 = Delete From Array(array=w755, length=1, index (col)=w749) -> (deleted portion=w751:dbl[][])  [unwired: 1 in, 1 out]
        n376 = Reshape Array(w751, 8 ("dimension size")) -> (w750:dbl[])
        n377 = call <vilib>:"Add State(s) to Queue__jki_lib_state_machine.vi"("State(s) in Front (\"\")"=w745, "State(s) in (\"\")"=w766) -> ("States Out"=w765:string)  [unwired: 13 in]
        n378 = Multiply(x=w743, y=w750) -> (x*y=w744:dbl[])
        "Currents" <- w744
        n379 = Bundle By Name(cluster=w763, "Read Data"=w744) -> (w762:T11)
        n380 = Index Array(array=w744, index="Channel") -> (element=→"Waveform Chart":dbl)
      }
      frame "Check for Rising Edge" {
        n381 = Unbundle By Name(w798) -> ("Read Data"=w796:dbl[], "Old Data"=w795:dbl[], "A Data"=w787:dbl[], "B Data"=w786:dbl[], "C Data"=w785:dbl[], "D Data"=w784:dbl[])
        n382 = local read "Max Len"() -> (w768:i32)
        n383 = Array Size(array=w787) -> (size(s)=w783:i32)
        n384 = Array Size(array=w786) -> (size(s)=w782:i32)
        n385 = Array Size(array=w785) -> (size(s)=w781:i32)
        n386 = Array Size(array=w784) -> (size(s)=w780:i32)
        n387 = Build Array(w783, w782, w781, w780) -> (w779:i32[])
        n388 = In Range and Coerce(upper limit=w768, x=w779, lower limit=0 ("Max Len of Cyc")) -> (In Range?=w778:bool[])  [unwired: 1 out]
        n389 = Not(x=w778) -> (.not. x?=w777:bool[])
        n390 = Less Or Equal?(x=w795, y="Off On Threshold") -> (x <= y?=w794:bool[])
        n391 = Greater?(x=w796, y="Off On Threshold") -> (0:w793:bool[])
        n392 = global read "Globals SS.vi" "A L1 Index"() -> (w791:i32)
        n393 = global read "Globals SS.vi" "B L1 index"() -> (w790:i32)
        n394 = global read "Globals SS.vi" "C L1 index"() -> (w789:i32)
        n395 = global read "Globals SS.vi" "D L1 index"() -> (w788:i32)
        n396 = And(x=w794, y=w793) -> (x .and. y?=w792:bool[])
        n397 = Index Array(array=w792, index #1=w791, index #2=w790, index #3=w789, index #4=w788) -> (element #1=w776:bool, element #2=w775:bool, element #3=w774:bool, element #4=w773:bool)
        n398 = Build Array(w776, w775, w774, w773) -> (w772:bool[])
        n399 = Compound Arithmetic op=AND(w772, w777) -> (w771:bool[])
        n400 = Bundle By Name(cluster=w798, "Old Data"=w796, "Rise"=w771) -> (w797:T11)
        n401 = call "WILT Rising Edge Latch.vi"("S Rising Edge"=w771) -> ()  [unwired: 10 in, 1 out]
        n402 = call <vilib>:"Add State(s) to Queue__jki_lib_state_machine.vi"("State(s) in (\"\")"=w801) -> ("States Out"=w800:string)  [unwired: 14 in]
      }
      frame "Add Data:A" {
        n403 = Unbundle By Name(w819) -> ("Read Data"=w815:dbl[], "A Data"=w813:dbl[], "A Data2"=w812:dbl[], "Alatch"=w811:bool, "Rise"=w805:bool[])
        n404 = Array To Cluster(array=w805) -> (cluster=w810:T12)
        n405 = local read "Max Len"() -> (w802:i32)
        n406 = global read "Globals SS.vi" "A L1 Index"() -> (w817:i32)
        n407 = global read "Globals SS.vi" "A L2 Index"() -> (w816:i32)
        n408 = Unbundle(w810) -> ("Rise[0]"=w809:bool)  [unwired: 3 out]
        n409 = Index Array(array=w815, index #1=w817, index #2=w816) -> (element #1=w808:dbl, element #2=w807:dbl)
        n410 = Or(x=w809, y=w811) -> (x .or. y?=w806:bool)
        n411 = case shown="True" w806 {
          tunnel: w809 -> [_ w829]
          tunnel: w813 -> [w825 w834]
          tunnel: [w825 w833] -> w804
          tunnel: w808 -> [_ w832]
          tunnel: [w824 w831] -> w803
          tunnel: w812 -> [w824 w830]
          tunnel: w807 -> [_ w828]
          tunnel: w802 -> [_ w827]
          tunnel: [w823 TRUE ("Alatch")] -> w814
          tunnel: w811 -> [w823 _]
          frame False {
          }
          frame True {
            n412 = call "WILT Add val to Array w Limit.vi"("size limit"=w827, "Value"=w828, "Array In"=w830, "Init?"=w829) -> ("Array  Out"=w831:dbl[])  [unwired: 7 in]
            n413 = call "WILT Add val to Array w Limit.vi"("size limit"=w827, "Value"=w832, "Array In"=w834, "Init?"=w829) -> ("Array  Out"=w833:dbl[])  [unwired: 7 in]
          }
        }
        n414 = local write "A Data"(w804) -> ()
        n415 = local write "A Data 2"(w803) -> ()
        n416 = Bundle By Name(cluster=w819, "Alatch"=w814, "A Data"=w804, "A Data2"=w803) -> (w818:T11)
        n417 = call <vilib>:"Add State(s) to Queue__jki_lib_state_machine.vi"("State(s) in (\"\")"=w822) -> ("States Out"=w821:string)  [unwired: 14 in]
      }
      frame "Add Data:B" {
        n418 = Unbundle By Name(w852) -> ("Read Data"=w848:dbl[], "B Data"=w846:dbl[], "B Data2"=w845:dbl[], "Blatch"=w844:bool, "Rise"=w839:bool[])
        n419 = Array To Cluster(array=w839) -> (cluster=w843:T12)
        n420 = global read "Globals SS.vi" "B L1 index"() -> (w850:i32)
        n421 = global read "Globals SS.vi" "B L2 index"() -> (w849:i32)
        n422 = Unbundle(w843) -> ("Rise[1]"=w838:bool)  [unwired: 3 out]
        n423 = Index Array(array=w848, index #1=w850, index #2=w849) -> (element #1=w842:dbl, element #2=w841:dbl)
        n424 = local read "Max Len"() -> (w835:i32)
        n425 = Or(x=w838, y=w844) -> (x .or. y?=w840:bool)
        n426 = case shown="True" w840 {
          tunnel: w838 -> [_ w862]
          tunnel: w846 -> [w858 w867]
          tunnel: [w858 w866] -> w837
          tunnel: w842 -> [_ w865]
          tunnel: [w857 w864] -> w836
          tunnel: w845 -> [w857 w863]
          tunnel: w841 -> [_ w861]
          tunnel: w835 -> [_ w860]
          tunnel: [w856 TRUE ("Alatch")] -> w847
          tunnel: w844 -> [w856 _]
          frame False {
          }
          frame True {
            n427 = call "WILT Add val to Array w Limit.vi"("size limit"=w860, "Value"=w861, "Array In"=w863, "Init?"=w862) -> ("Array  Out"=w864:dbl[])  [unwired: 7 in]
            n428 = call "WILT Add val to Array w Limit.vi"("size limit"=w860, "Value"=w865, "Array In"=w867, "Init?"=w862) -> ("Array  Out"=w866:dbl[])  [unwired: 7 in]
          }
        }
        n429 = Bundle By Name(cluster=w852, "Blatch"=w847, "B Data"=w837, "B Data2"=w836) -> (w851:T11)
        n430 = local write "B Data 2"(w836) -> ()
        n431 = local write "B Data"(w837) -> ()
        n432 = call <vilib>:"Add State(s) to Queue__jki_lib_state_machine.vi"("State(s) in (\"\")"=w855) -> ("States Out"=w854:string)  [unwired: 14 in]
      }
      frame "Add Data:C" {
        n433 = Unbundle By Name(w885) -> ("Read Data"=w881:dbl[], "C Data"=w879:dbl[], "C Data2"=w878:dbl[], "Clatch"=w877:bool, "Rise"=w872:bool[])
        n434 = Array To Cluster(array=w872) -> (cluster=w876:T12)
        n435 = global read "Globals SS.vi" "C L1 index"() -> (w883:i32)
        n436 = global read "Globals SS.vi" "C L2 index"() -> (w882:i32)
        n437 = Unbundle(w876) -> ("Rise[2]"=w871:bool)  [unwired: 3 out]
        n438 = Index Array(array=w881, index #1=w883, index #2=w882) -> (element #1=w875:dbl, element #2=w874:dbl)
        n439 = Or(x=w871, y=w877) -> (x .or. y?=w873:bool)
        n440 = local read "Max Len"() -> (w868:i32)
        n441 = case shown="True" w873 {
          tunnel: w871 -> [_ w895]
          tunnel: w879 -> [w891 w900]
          tunnel: [w891 w899] -> w870
          tunnel: w875 -> [_ w898]
          tunnel: [w890 w897] -> w869
          tunnel: w878 -> [w890 w896]
          tunnel: w874 -> [_ w894]
          tunnel: w868 -> [_ w893]
          tunnel: [w889 TRUE ("Alatch")] -> w880
          tunnel: w877 -> [w889 _]
          frame False {
          }
          frame True {
            n442 = call "WILT Add val to Array w Limit.vi"("size limit"=w893, "Value"=w894, "Array In"=w896, "Init?"=w895) -> ("Array  Out"=w897:dbl[])  [unwired: 7 in]
            n443 = call "WILT Add val to Array w Limit.vi"("size limit"=w893, "Value"=w898, "Array In"=w900, "Init?"=w895) -> ("Array  Out"=w899:dbl[])  [unwired: 7 in]
          }
        }
        n444 = local write "C Data 2"(w869) -> ()
        n445 = Bundle By Name(cluster=w885, "Clatch"=w880, "C Data"=w870, "C Data2"=w869) -> (w884:T11)
        n446 = local write "C Data"(w870) -> ()
        n447 = call <vilib>:"Add State(s) to Queue__jki_lib_state_machine.vi"("State(s) in (\"\")"=w888) -> ("States Out"=w887:string)  [unwired: 14 in]
      }
      frame "Add Data:D" {
        n448 = Unbundle By Name(w918) -> ("Read Data"=w914:dbl[], "D Data"=w912:dbl[], "D Data2"=w911:dbl[], "Dlatch"=w910:bool, "Rise"=w905:bool[])
        n449 = Array To Cluster(array=w905) -> (cluster=w909:T12)
        n450 = global read "Globals SS.vi" "D L1 index"() -> (w916:i32)
        n451 = global read "Globals SS.vi" "D L2 index"() -> (w915:i32)
        n452 = Unbundle(w909) -> ("Rise[3]"=w904:bool)  [unwired: 3 out]
        n453 = Index Array(array=w914, index #1=w916, index #2=w915) -> (element #1=w908:dbl, element #2=w907:dbl)
        n454 = Or(x=w904, y=w910) -> (x .or. y?=w906:bool)
        n455 = local read "Max Len"() -> (w901:i32)
        n456 = case shown="True" w906 {
          tunnel: w904 -> [_ w928]
          tunnel: w912 -> [w924 w933]
          tunnel: [w924 w932] -> w903
          tunnel: w908 -> [_ w931]
          tunnel: [w923 w930] -> w902
          tunnel: w911 -> [w923 w929]
          tunnel: w907 -> [_ w927]
          tunnel: w901 -> [_ w926]
          tunnel: [w922 TRUE ("Alatch")] -> w913
          tunnel: w910 -> [w922 _]
          frame False {
          }
          frame True {
            n457 = call "WILT Add val to Array w Limit.vi"("size limit"=w926, "Value"=w931, "Array In"=w933, "Init?"=w928) -> ("Array  Out"=w932:dbl[])  [unwired: 7 in]
            n458 = call "WILT Add val to Array w Limit.vi"("size limit"=w926, "Value"=w927, "Array In"=w929, "Init?"=w928) -> ("Array  Out"=w930:dbl[])  [unwired: 7 in]
          }
        }
        n459 = Bundle By Name(cluster=w918, "Dlatch"=w913, "D Data"=w903, "D Data2"=w902) -> (w917:T11)
        n460 = local write "D Data 2"(w902) -> ()
        n461 = local write "D Data"(w903) -> ()
        n462 = call <vilib>:"Add State(s) to Queue__jki_lib_state_machine.vi"("State(s) in (\"\")"=w921) -> ("States Out"=w920:string)  [unwired: 14 in]
      }
    }
  }
  n463 = property on="Stop" class="Bool (strict)"("Val(Sgnl)"=w3) -> ()  [unwired: 2 in, 2 out]
